vi "FocalMainV2.vi"() -> ()   [LabVIEW 2018]
uses:
  Clusters/FileDataChannel.ctl
  Clusters/BladePitchMode.ctl
  Clusters/GenMode.ctl
  Clusters/IndicatorScale.ctl
  Clusters/SimulationConstants.ctl
  Clusters/IOSignals.ctl
  <vilib>/Platform/TimedLoop/XDataNode/timing_clust.ctl
  <vilib>/Platform/TimedLoop/XDataNode/nitl_modes.ctl
  <vilib>/Platform/TimedLoop/XDataNode/wakeup.ctl
  Clusters/ArrayPairs.ctl
  Clusters/SwapArrayCluster.ctl
  Clusters/ElmoState.ctl
  Clusters/CtrlSignals.ctl
  Clusters/ScalingEnum.ctl
  Clusters/AnemometerData.ctl
  Clusters/RoscoParams.ctl
  Clusters/GenCtrl.ctl
  Clusters/PitchCtrl.ctl
  <vilib>/Instr/_visa.llb/VISA Configure Serial Port (Instr).vi
  SubVIs/InsertIntoArray_v2.vi
  <vilib>/platform/TimedLoop/XDataNode/XDataNode.xnode
  <vilib>/Platform/TimedLoop/XDataNode/XDNodeRunTimeDep.lvlib
  <resource>/objmgr/IndComECAT.rc
  usr/local/lib/libCallROSCO.so
  <vilib>/ptbypt/NI_PtbyPt.lvlib
panel:
  out "anemoRefU_m_s":dbl
  out "RS232 loop late?":bool
  in  "Fan Setpoint (%)":dbl format="%#_13g"
  out "Setpoint file loaded":path
  in  "Ctrl Mode":enum32{"Manual", "FromFile"}(radio)
  in  "Setpoint file name":string="setpointsVelTestA.txt"
  in  "Reload File":bool
  in  "windSpeed_m_s":dbl format="%#_13g"
  out "towerBotMy":dbl
  out "Current Setting":dbl[](array[numeric])
  in  "Commit":bool
  in  "Clear Faults":bool
  in  "Enable Fans":bool
  in  "Turn Fans On":bool
  out "Fy":dbl format="%#_5g"
  out "Fx":dbl
  out "PLC read errors":string
  out "PLC read/write late?":bool
  out "PLC Read Error":bool
  out "Axis 3 Homing":bool
  out "Axis 2 Homing":bool
  out "Axis 1 Homing":bool
  in  "Home Blades (x3)":bool
  out "Axis 3 Homed":bool
  out "Axis 2 Homed":bool
  out "Axis 1 Homed":bool
  out "SimulationConst":T1={"nGear"=1.0, "rotorRadius"=120.0, "numBlades"=3, "scaleFactor"=70.0, "roscoInitMinSpeed_rad_s"=0.5, "roscoInitMinTorqueFS_Nm"=1000000.0, "beckhoff16bit"=1000000.0, "beckhoff24BitExt"=7812500, "rotorTorqueScale_Nm_V"=5.0, "rotorTorqueOfst_Nm"=2.0, "rangeEL3104V"=10.0, "nacelleAccELM3604V"=1.25, "nacelleAccScaleX_m_s2_V"=0.0673, "nacelleAccOfstX_m_s2"=0.0055, "nacelleAccScaleY_m_s2_V"=0.0672, "nacelleAccOfstY_m_s2"=0.0049, "nacelleAccScaleZ_m_s2_V"=0.0677, "nacelleAccOfstZ_m_s2"=0.0087, "cyberGearRatio"=0.5, "cyberLinesPerRev"=0.5, "cyberRatedTorque"=0.5, "towerTopForceScale"=0.5, "towerTopTorqueScale"=0.5, "plcSetpointScaling_norm2VFD"=0.5, "towerBotScaleMy_Nm_V"=0.5, "towerBotOfstMy_Nm"=0.5, "towerTopScaleXaxis_N_V"=0.5, "towerTopOfstXaxis_N"=0.5, "towerTopScaleYaxis_N_V"=0.5, "towerTopOfstYaxis_N"=0.5, "pitchFlagOffset_deg"=0.5, "anemWindSpeedScaleU_m_s_m_s"=0.5, "anemWindSpeedOfstU_m_s"=0.5, "anemWindSpeedScaleV_m_s_m_s"=0.5, "anemWindSpeedOfstV_m_s"=0.5, "anemWindSpeedScaleW_m_s_m_s"=0.5, "anemWindSpeedOfstW_m_s"=0.5, "anemWindSpeedScaleTSI1_m_s_V"=0.5, "anemWindSpeedOfstTSI1_m_s"=0.5} {"beckhoff16bit" format="%x"}
  out "nacelleAccZ (m/s2)":dbl
  out "nacelleAccY (m/s2)":dbl
  out "nacelleAccX (m/s2)":dbl
  out "Disk > 2GB free?":bool
  out "Current OP mode":T2
  in  "IndicatorScale":T3
  in  "DISCON.IN file":string="DISCON-UMaineSemi.IN"
  in  "Cp/Ct/Cq file":string="Cp_Ct_Cq.IEA15MW.txt"
  out "Torque sine period FS (Nm)":dbl format="%.2g"
  out "Torque sine amp FS (Nm)":dbl format="%.2g"
  out "Torque sine mean FS (Nm)":dbl format="%.2g"
  out "Ramp time FS (s)":dbl format="%.2g"
  out "Ramp target vel FS (rpm)":dbl format="%.2g"
  out "Const. vel setpoint FS (rpm)":dbl format="%.2g"
  out "From File RotSpd FS (rpm)":dbl
  out "From File Pitch FS (deg)":dbl
  out "Exp time FS (s)":dbl format="%5.2f"
  in  "Commit gen settings":bool
  out "Current OP mode":T4
  in  "Commit pitch settings":bool
  in  "Start / Stop Run":bool
  out "Speed Setpoint (rpm)":dbl(knob)=7.068579725455493e-05 scale=0.0..20.0
  out "Pitch Blade 3 (deg)":dbl
  out "Pitch Bade 2 (deg)":dbl
  out "Pitch Blade 1 (deg)":dbl
  out "Pitch Setpoint (deg)":dbl
  out "Torque sine period MS (Nm)":dbl format="%.2g"
  out "Torque sine amp MS (Nm)":dbl format="%#.2g"
  in  "Torque sine period (s)":dbl=100.0
  in  "Torque sine amp (MNm)":dbl
  out "Torque sine mean MS (Nm)":dbl format="%.2g"
  in  "Torque mean (MNm)":dbl
  out "Ramp time MS (s)":dbl format="%.2g"
  out "Ramp target vel MS (rpm)":dbl format="%.2g"
  out "Const. vel setpoint MS (rpm)":dbl format="%.2g"
  in  "Ramp time (s)":dbl=100.0
  in  "Ramp target vel (rpm)":dbl=1.0
  in  "Const. vel (rpm)":dbl
  out "Current Const. (deg)":dbl
  in  "Next OP mode":T2
  in  "Next Const. (deg)":dbl=10.0
  in  "Next OP mode":T4
  in  "Wind Est. u(t=0)":dbl=5.0
  out "Exp. Time MS (s)":dbl format="%5.1f"
  out "Output file Name":string
  out "State logic late?":bool
  out "Axis 3 Fault":bool
  out "Axis 3 Warning":bool
  out "Axis 2 Fault":bool
  out "Axis 2 Warning":bool
  out "Axis 1 Fault":bool
  out "Axis 1 Warning":bool
  out "Axis 3 Operational":bool
  out "Axis 2 Operational":bool
  out "Axis 1 Operational":bool
  out "Pitch Axis 3 State":string
  out "Pitch Axis 2 State":string
  out "Pitch Axis 1 State":string
  in  "Clear Pitch Actuator Faults (x3)":bool
  in  "Enable Pitch Actuators (x3)":bool
  out "Generator Operational":bool
  in  "Clear Accelnet Faults":bool
  in  "Enable Accelnet":bool
  out "Generator Fault":bool
  out "Generator Warning":bool
  out "Main generator state":string
  out "Rosco Failed?":bool
  out "Torque Cell":dbl(knob) scale=0.0..25.0
  out "Actual Speed MS (rpm)":dbl(knob)=7.068579725455493e-05 scale=0.0..20.0
  in  "?":T5(tab)
  out "Accel":dynamicdata(graph)
  out "Generator Speed":dynamicdata(graph)
  out "Rotor Loads":dynamicdata(graph)
  out "Pitch":dynamicdata(graph)
  in  "Sample":bool
  in  "Apply Ofst":bool
  out "FxMean":dbl format="%0.2f"
  out "FyMean":dbl format="%0.2f"
  out "MyMean":dbl format="%0.2f"
  out "DISCON.IN Contents":string
  out "Rosco Interface Current Message":string
  out "ROSCO DISCON.In file used":string
  out "ROSCO CpCqCt File used":string
  out "ROSCO out file used":string
  out "Test sum":sgl
  out "error out":errorcluster
  out "aviFAIL":i32
  out "Rosco Interface First Message":string
  out "Rosco Setpoint (Nm) - MS":dbl(knob) scale=0.0..10.0
  out "OUT_ROTSP":dbl
  out "OUT_AEROTQ":dbl
  out "Rosco Pitch Setpoint (rad)":dbl(knob) scale=0.0..10.0
  out "WE ROSCO":dbl
  out "avrSWAP":sgl[](array[numeric])
  out "Setpoints":dbl[][](array[numeric])
  out "Time index":i32
  out "Loop duration (ms)":i64
  in  "Pitch Max Vel Change (rpm/min) - FS":dbl=10.0
  in  "Pitch Max Vel (rpm) - FS":dbl=1.0
  in  "Pitch Homing Vel  (rpm) - FS":dbl=0.3
  in  "Pitch P-Gain":dbl=5.0
  in  "Max Vel (rpm)  -FS":dbl=14.0
  in  "Velocity Ctrl P-Gain":dbl=0.14
  in  "Velocity Ctrl I-Gain":dbl=3.0
  in  "Torque Ctrl FF Gain":dbl=1.15
  in  "Torque Ctrl I-Gain":dbl=5.0
  in  "Torque Ctrl P-Gain":dbl=0.05
  in  "Max Torque (MNm) - FS":dbl=25.0
  out "Pitch axis 3 ctrl word":u16 format="%x"
  out "Pitch axis 2 ctrl word":u16 format="%x"
  out "RT Loop Duration":i64
  out "Control Mode - Main Gen":u8
  out "WriteSDO Abort - Main Gen":u32
  out "ReadSDO Abort - Main Gen":u32
  out "Gen ctrl word":u16 format="%x"
  out "Pitch axis 1 ctrl word":u16 format="%x"
  out "Graphics Update t (s)":dbl format="%.1f"
  out "Effective graphics rate (ms)":dbl format="%#.1f"
  out "WriteSDO Abort - Pitch 1":u32
  out "ReadSDO Abort - Pitch 1":u32
  out "Control Mode - Pitch 1":u8
  out "Torque RAW (V)":dbl
  out "Torque Sensor (Nm) - NOT scaled":dbl(knob) scale=-2.0..2.0
  out "Free GB disk":dbl
  out "WriteSDO Abort - Pitch 2":u32
  out "Control Mode - Pitch 2":u8
  out "ReadSDO Abort - Pitch 2":u32
  out "WriteSDO Abort - Pitch 3":u32
  out "Control Mode - Pitch 3":u8
  out "ReadSDO Abort - Pitch 3":u32
  out "MotorDemandTorque_Nm":dbl(knob) scale=-2.0..2.0
  out "MotorCurrentTorq (Nm)":dbl(knob) scale=-2.0..2.0
  out "Axis 1 HomePos (rad)":dbl
  out "Axis 2 HomePos (rad)":dbl
  out "Axis 3 HomePos (rad)":dbl
  out "Init error":errorcluster
  out "Setpoint read error":string
  out "Torque Setpoint":dbl(knob) scale=0.0..35.0
  out "Power (MW)":dbl(slide) scale=0.0..10.0 scale format="%.2f"
  out "FIFO Loop Late?":bool
  in  "Base filename":string="rosco-tests"
  out "Writing":bool
  in  "?":T6
  out "#RT FIFO":u32
  in  "Stop LabVIEW":bool
  out "cRio Time(s)":dbl format="%6.1f"
  out "RT Loop Late?":bool
  # "FOCAL Campaign 1 - V2.1"
  # "ROSCO OK?"
  # "GENERATOR ENABLE"
  # "BLADE PITCH"
  # "WIND MACHINE CONTROL"
  # "EXPERIMENT CONTROL"
  # "GENERATOR SETPOINT CTRL"
  # "PITCH ACTUATORS CONTROL"
  # "Nacelle Acceleration"
  # "TowerTop 3DOF"
  # "Blade1"
  # "Blade2"
  # "Blade3"
  # "Current values"
  # "Operational"
  # "Enter NEXT values (FS)"
  # "FS"
  # "MS"
  # "Homing"
  # "Homed"
  # "Warning"
  # "Error"
  # "TowerBot My"
  # "Fan 1"
  # "Time"
  # "Pitch"
  # "RotSpd"
  # "Fan 20"
  # "Fan 30"
  # "Fan 10"
  # "PI for Torque Ctrl"
  # "PI for Velocity Ctrl"
  # "PI for Pitch Ctrl"
  # "Main Gen Limits"
  # "Pitch limits"
  # "PITCH AXIS 1"
  # "PITCH AXIS 2"
  # "PITCH AXIS 3"
  # "TOWER TOP 6DOF"
  # "SYSTEM"
  # "GENERATOR"
  # "TORQUE SENSOR"
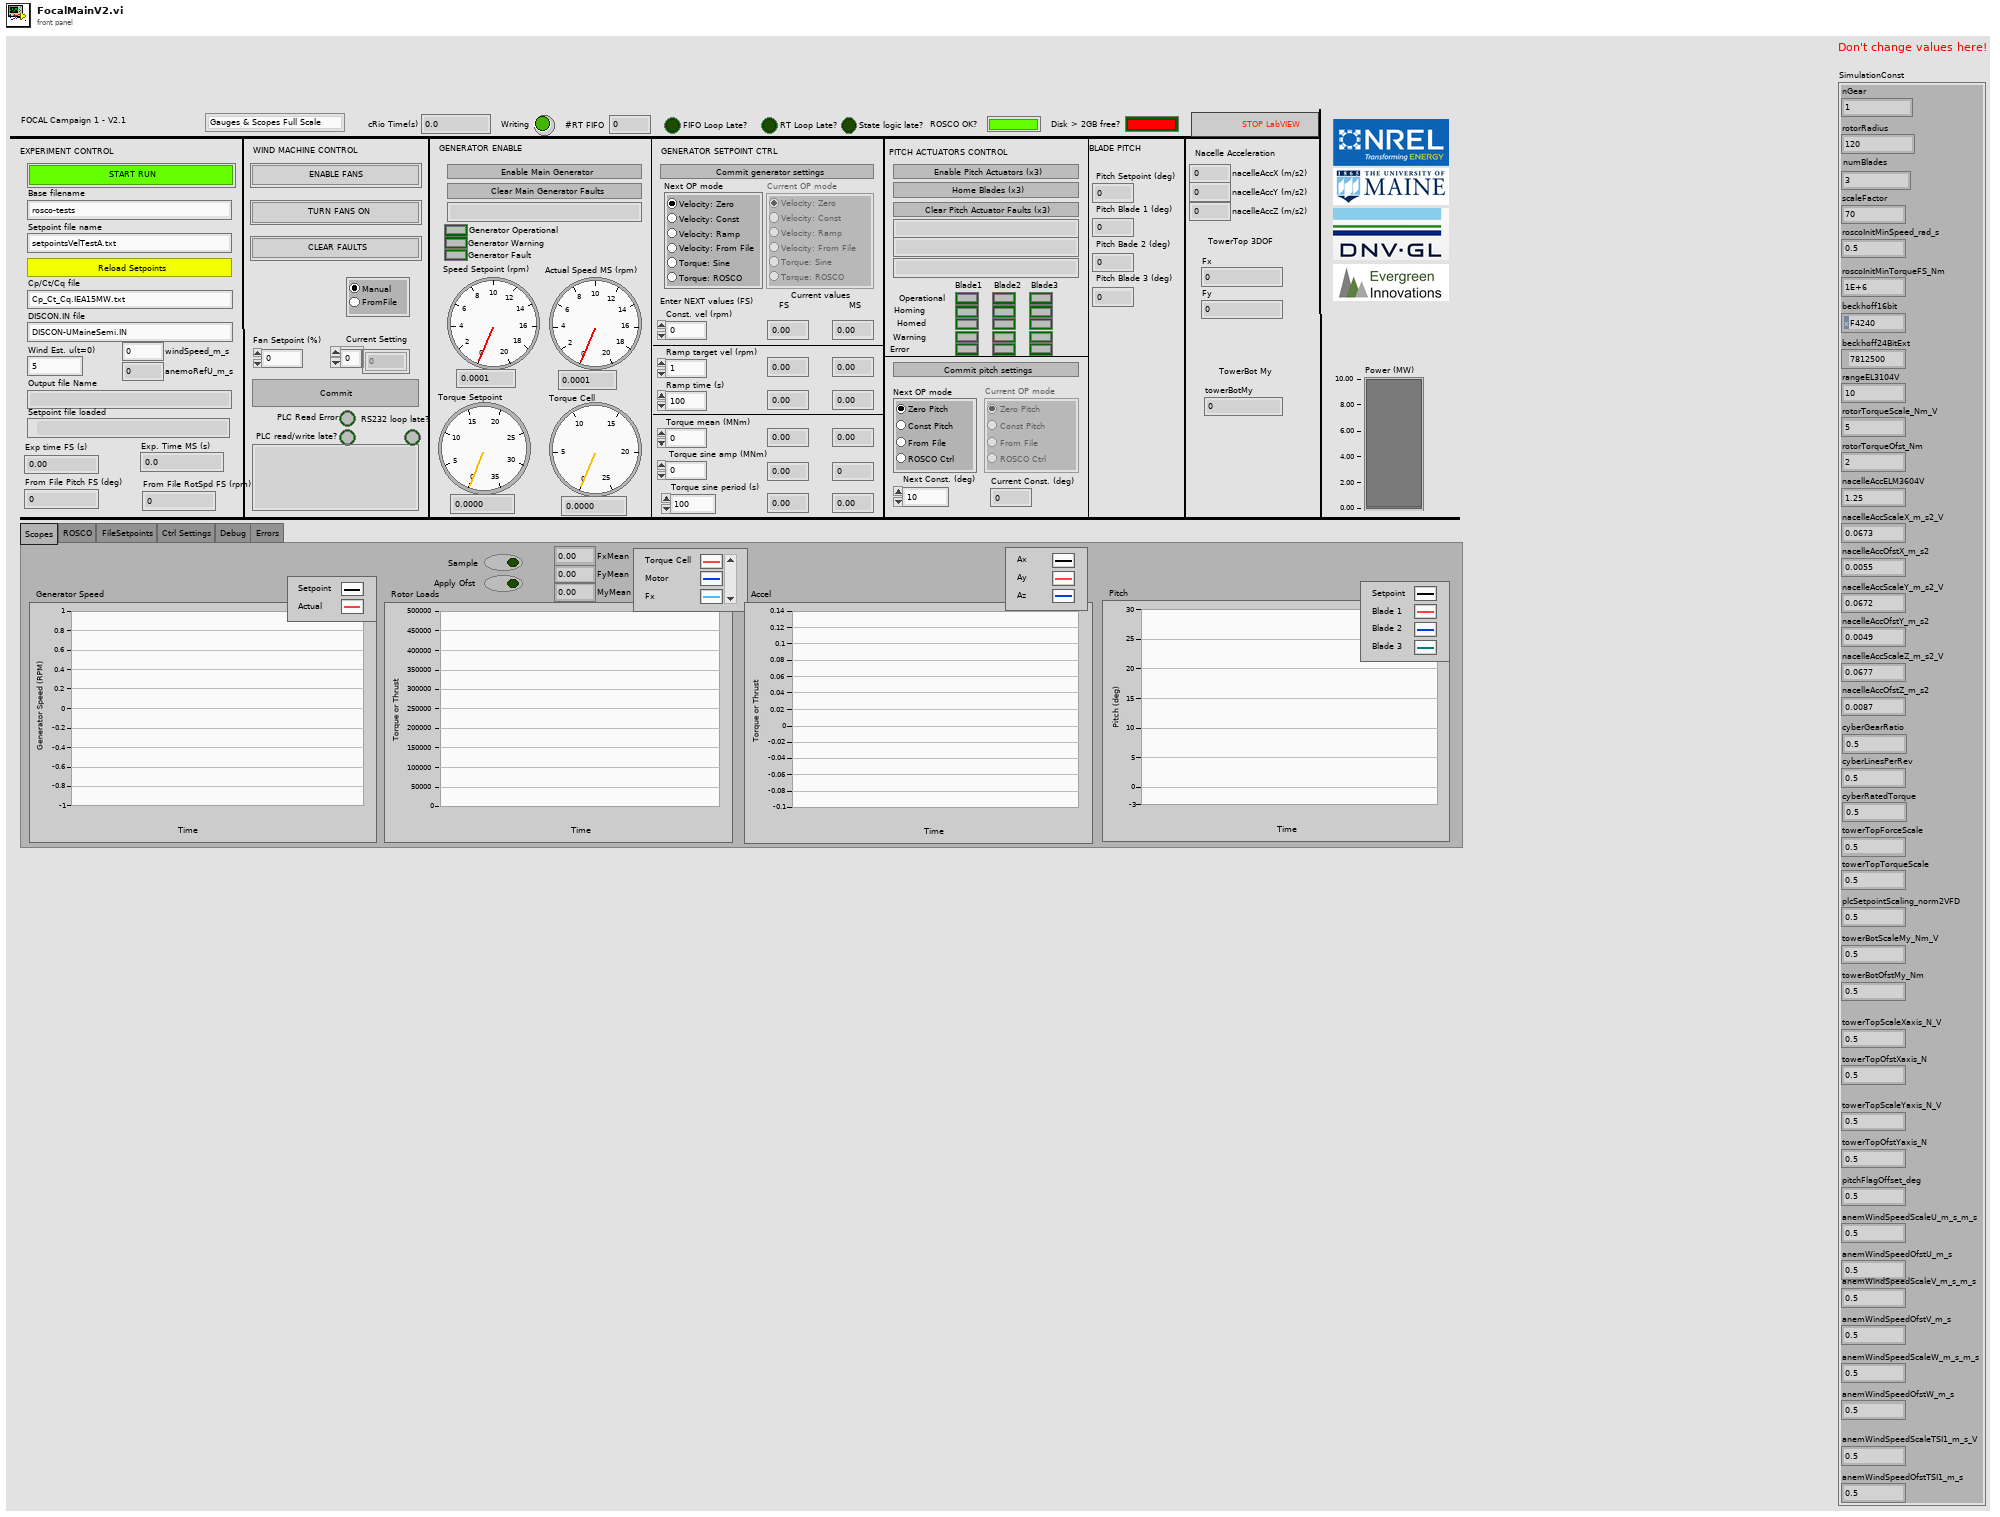
[diagram p1: front panel]
types:
  T1 = typedef "SimulationConstants.ctl" = cluster{"nGear":dbl, "rotorRadius":sgl, "numBlades":i32, "scaleFactor":dbl, "roscoInitMinSpeed_rad_s":dbl, "roscoInitMinTorqueFS_Nm":dbl, "beckhoff16bit":dbl, "beckhoff24BitExt":i32, "rotorTorqueScale_Nm_V":dbl, "rotorTorqueOfst_Nm":dbl, "rangeEL3104V":dbl, "nacelleAccELM3604V":dbl, "nacelleAccScaleX_m_s2_V":dbl, "nacelleAccOfstX_m_s2":dbl, "nacelleAccScaleY_m_s2_V":dbl, "nacelleAccOfstY_m_s2":dbl, "nacelleAccScaleZ_m_s2_V":dbl, "nacelleAccOfstZ_m_s2":dbl, "cyberGearRatio":dbl, "cyberLinesPerRev":dbl, "cyberRatedTorque":dbl, "towerTopForceScale":dbl, "towerTopTorqueScale":dbl, "plcSetpointScaling_norm2VFD":dbl, "towerBotScaleMy_Nm_V":dbl, "towerBotOfstMy_Nm":dbl, "towerTopScaleXaxis_N_V":dbl, "towerTopOfstXaxis_N":dbl, "towerTopScaleYaxis_N_V":dbl, "towerTopOfstYaxis_N":dbl, "pitchFlagOffset_deg":dbl, "anemWindSpeedScaleU_m_s_m_s":dbl, "anemWindSpeedOfstU_m_s":dbl, "anemWindSpeedScaleV_m_s_m_s":dbl, "anemWindSpeedOfstV_m_s":dbl, "anemWindSpeedScaleW_m_s_m_s":dbl, "anemWindSpeedOfstW_m_s":dbl, "anemWindSpeedScaleTSI1_m_s_V":dbl, "anemWindSpeedOfstTSI1_m_s":dbl}
  T2 = typedef "GenMode.ctl" = enum32{"Velocity: Zero", "Velocity: Const.", "Velocity: Ramp", "Velocity: From File", "Torque: Sine", "Torque: ROSCO"}
  T3 = typedef "IndicatorScale.ctl" = enum16{"Gauges & Scopes Full Scale", "Gauges & Scopes Model Scale"}
  T4 = typedef "BladePitchMode.ctl" = enum32{"Zero pitch", "Const pitch", "From File", "ROSCO Ctrl"}
  T5 = enum32{"Scopes", "ROSCO", "FileSetpoints", "Ctrl Settings", "Debug", "Errors"}
  T6 = typedef "FileDataChannel.ctl" = cluster{"dataTime_s":dbl, "dataLoopCounter":dbl, "anemoRefU_m_s":dbl, "anemoRefV_m_s":dbl, "anemoRefW_m_s":dbl, "rotorTorque_Nm":dbl, "towerTopFx_N":dbl, "towerTopFy_N":dbl, "towerBotMy_Nm":dbl, "accelNacelleAx_m_s2":dbl, "accelNacelleAy_m_s2":dbl, "accelNacelleAz_m_s2":dbl, "genSpeed_rad_s":dbl, "genTorque_Nm":dbl, "genStatus":dbl, "pitch1Position_rad":dbl, "pitch1Velocity_rad_s":dbl, "pitch1Status":dbl, "pitch2Position_rad":dbl, "pitch2Velocity_rad_s":dbl, "pitch2Status":dbl, "pitch3Position_rad":dbl, "pitch3Velocity_rad_s":dbl, "pitch3Status":dbl, "genUserOpMode":dbl, "pitchUserOpMode":dbl, "torqueSetpointRosco_Nm":dbl, "pitchSetpointRosco_rad":dbl, "fan1Setpt_%":dbl, "genTorqueSetpointActual_Nm":dbl, "pitchSetpointActual_rad":dbl, "genVelSetpoint_radps":dbl, "genPosition_rad":dbl, "towerTopFz_N":dbl, "towerTopMx_Nm":dbl, "towerTopMy_Nm":dbl, "towerTopMz_Nm":dbl}
  T7 = typedef "CtrlSignals.ctl" = cluster{"Enable":bool, "On":bool, "Reset Fault":bool}
  T8 = typedef "ElmoState.ctl" = cluster{"Elmo Operational":bool, "Elmo Warning":bool, "Elmo Fault":bool, "Blade Homed":bool, "Blade Homing":bool, "HomePos (rad)":dbl}
  T9 = typedef "ArrayPairs.ctl" = cluster{"iStatus":T10, "TIME":T10, "DT":T10, "Blade1PitchPos_rad":T10, "VS_MECHGENPWR":T10, "VS_GENPWR":T10, "GEN_SPEED":T10, "ROTOR_SPEED":T10, "GENTQMEAS":T10, "Y_M":T10, "HORWINDV":T10, "ROOTMOOP1":T10, "ROOTMOOP2":T10, "Blade2PitchPos_rad":T10, "Blade3PitchPos_rad":T10, "ROOTMOOP3":T10, "AVCMSG_SIZE":T10, "INFILE_SIZE ":T10, "OUTFILE_SIZE ":T10, "FA_ACC":T10, "NUM_BLADES":T10, "BladePitchSetpoint_rad":T10, "TorqueSetpoint_Nm":T10, "OUT_AEROTQ":T10, "Out.RotSpeed ":T10, "Out.DEBUG":T10}
  T10 = typedef "SwapArrayCluster.ctl" = cluster{"Index":i32, "Value":dbl}
  T11 = typedef "IOSignals.ctl" = cluster{"mainGenPosition (rad)":dbl, "motorCurrentTorq (Nm)":dbl, "mainGenVelocity (rad/s)":dbl, "mainGenStatus":u16, "pitch1Position (rad)":dbl, "pitch1Velocity (rad/s)":dbl, "pitch1Status":u16, "pitch2Position (rad)":dbl, "pitch2Velocity (rad/s)":dbl, "pitch2Status":u16, "pitch3Position (rad)":dbl, "pitch3Velocity (rad/s)":dbl, "pitch3Status":u16, "torqueSensor (Nm)":dbl, "nacelleAccX (m/s2)":dbl, "nacelleAccY (m/s2)":dbl, "nacelleAccZ (m/s2)":dbl, "pitch1HomeFlag":bool, "pitch2HomeFlag":bool, "pitch3HomeFlag":bool, "towerTopFx (N)":dbl, "towerTopFy (N)":dbl, "towerBotMy (Nm)":dbl, "anemoRefU_m_s":dbl, "anemoRefV_m_s":dbl, "anemoRefW_m_s":dbl}
  T12 = enum16{"open", "replace", "create", "open or create", "replace or create", "replace or create with confirmation"}
  T13 = typedef "RoscoParams.ctl" = cluster{"avrSWAP":dbl[], "aviFAIL":i32, "currentMsg":string, "ReturnValue":i32, "disconInFileName":string, "outFileName":string, "firstMsg":string}
  T14 = typedef "XDNodeRunTimeDep.lvlib/timing_clust.ctl" = cluster{"Expected End [f-1]":u64, "Actual End [f-1]":u64, "Finished Late? [f-1]":bool, "Expected End [i-1]":u64, "Actual End [i-1]":u64, "Finished Late? [i-1]":bool, "Expected Start [i]":u64, "Actual Start [i]":u64, "Expected Start [f]":u64, "Actual Start [f]":u64, "Source Name":string, "Structure Name":string, "Period":i64, "Deadline":i64, "Offset":i64, "Start":i64, "Priority":i32, "Timeout":i32, "Mode":T15, "Wakeup Reason":T16, "Error":errorcluster, "Source Type":string, "Secondary Source Type":string, "Global End Time":u64, "Global Start Time":u64, "Frame Duration":u64, "Iteration Duration":u64, "Assigned CPU":i32, "I/O Scan Engine Mode":u32}
  T15 = typedef "XDNodeRunTimeDep.lvlib/nitl_modes.ctl" = enum32{"No Change", "Process missed periods, maintain original phase", "Discard missed periods, maintain original phase", "Process missed periods, ignore original phase", "Discard missed periods, ignore original phase"}
  T16 = typedef "XDNodeRunTimeDep.lvlib/wakeup.ctl" = enum32{"Normal", "Aborted", "Asynchronous wakeup", "Timing source error", "Timed loop error", "Timeout"}
  T17 = enum8{"Enabled", "Disabled", "Disabled and Grayed Out"}
  T18 = typedef "ScalingEnum.ctl" = enum16{"Model scale -> Full scale", "Full scale -> Model scale"}
  T19 = typedef "GenCtrl.ctl" = cluster{"Constant velocity setpoint (rpm)":dbl, "Ramp target velocity (rpm)":dbl, "Ramp time (s)":dbl, "Sine mean (Nm)":dbl, "Sine amp (Nm)":dbl, "Sine period (s)":dbl, "Torque Ctrl I-Gain":dbl, "Velocity Ctrl P-Gain":dbl, "Velocity Ctrl I-Gain":dbl, "Max Torque (Nm)":dbl, "GeneratorOn":bool, "Torque Ctrl P-Gain":dbl, "From file velocity (rpm)":dbl, "Generator operating mode":T2, "Max Vel (rpm)":dbl, "Torque Ctrl FF Gain":dbl}
  T20 = typedef "PitchCtrl.ctl" = cluster{"P-Gain":dbl, "Blade pitch operating mode":T4, "Constant setpoint (deg)":dbl, "I-Gain":dbl, "Pitch from File (deg)":dbl, "Homing vel (rpm)":dbl, "Max vel (rpm)":dbl, "Max vel change (rpm/min)":dbl}
  T21 = typedef "AnemometerData.ctl" = cluster{"Wind speed, U (m/s)":dbl, "Wind speed, V (m/s)":dbl, "Wind speed, W (m/s)":dbl}
  T22 = typedef "AccelnetState.ctl" = cluster{"State String":string, "Accelnet Warning":bool, "Accelnet Fault":bool, "Accelnet Operational":bool}
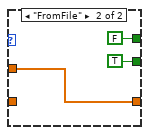
[diagram p5: hidden frame]
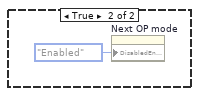
[diagram p12: hidden frame]
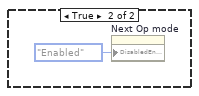
[diagram p13: hidden frame]
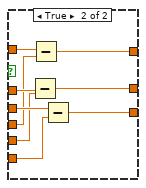
[diagram p15: hidden frame]
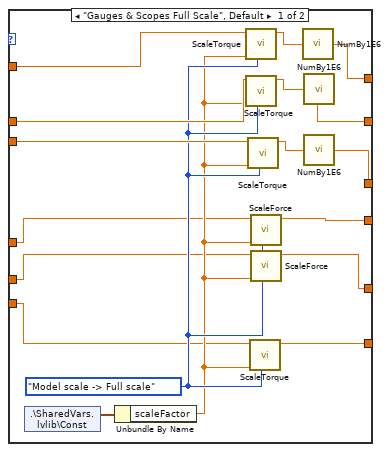
[diagram p17: hidden frame]
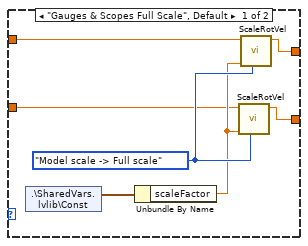
[diagram p18: hidden frame]
diagram:
  w2 = T7 {"Enable"=FALSE, "On"=FALSE, "Reset Fault"=FALSE}  # Ctrl State
  w10 = T7 {"Enable"=FALSE, "On"=FALSE, "Reset Fault"=FALSE}  # Current State
  w8 = errorcluster {"status"=FALSE, "code"=0, "source"=""}  # Error
  w20 = u16 10 items=["1.0"=10, "1.5"=15, "2.0"=20] ("stop bits (10: 1 bit)")
  w21 = u16 0 items=["None", "XON/XOFF", "RTS/CTS", "XON/XOFF & RTS/CTS", "DTR/DSR", "XON/XOFF & DTR/DSR"] ("flow control (0:none)")
  w74 = i64 2000 ("Period")
  # "Setpoint VFD"
  # "Current VFD read from PLC"
  # "Adjust this once we get a feeling for IO latency to/from the PLC"
  # "Runs at 64 Hz = 15.625ms = 15625 us"
  # "Manual Vel Set"
  # "Rotor Spd init"
  # "Blade Pitch init"
  # "Velocity Setpoint init"
  # "Time init"
  # "us -> s"
  # "in us"
  # "Init torque sine period"
  # "Init torque sine amp"
  # "Init torque mean"
  # "Init Ramp time"
  # "Init Ramp target vel"
  # "Init Const. Vel"
  # "Initial pitch"
  # "Code to remove"
  # "dt (s)"
  # "5ms = 200Hz"
  # "group name"
  n1 = flat-sequence {
    tunnel: [w123] -> w89
    tunnel: [w124] -> w88
    tunnel: [w116] -> w82
    tunnel: [w115] -> w81
    tunnel: [w102] -> w54
    tunnel: [w101] -> w53
    tunnel: [w100] -> w52
    tunnel: [w99] -> w51
    tunnel: w89 -> [w167]
    tunnel: w88 -> [w166]
    tunnel: w82 -> [w157]
    tunnel: w81 -> [w156]
    tunnel: [w153] -> w48
    tunnel: w54 -> [w144]
    tunnel: w53 -> [w143]
    tunnel: w52 -> [w133]
    tunnel: w51 -> [w132]
    tunnel: w48 -> [w177]
    tunnel: [w177] -> w47
    tunnel: [w225] -> w84
    tunnel: [w219] -> w92
    tunnel: [w212] -> w67
    tunnel: w47 -> [w212]
    tunnel: [w193] -> w56
    frame #0 {
      w100 = refnum<k21> "ni.var.io://NI-cRIO-9036-01B82934/EtherCAT Master/PitchBlade3" ("Slave Constant")
      w102 = refnum<k21> "ni.var.io://NI-cRIO-9036-01B82934/EtherCAT Master/PitchBlade2" ("Slave Constant")
      w116 = refnum<k21> "ni.var.io://NI-cRIO-9036-01B82934/EtherCAT Master/PitchBlade1" ("Slave Constant")
      w123 = refnum<k21> "ni.var.io://NI-cRIO-9036-01B82934/EtherCAT Master/MainGen" ("Slave Constant")
      # "Mode of operation for Pitch Blade 3"
      # "Mode of operation"
      # "8 = CSP \n9 = CSV\n10 = CST"
      # "Mode of operation for Pitch Blade 2"
      # "Mode of operation"
      # "8 = CSP \n9 = CSV\n10 = CST"
      # "Note: Operate in CST, and close velocity loop in LabVIEW when required"
      # "Mode of operation for Pitch Blade 1"
      # "Mode of operation for Main Gen"
      # "Mode of operation"
      # "8 = CSP \n9 = CSV\n10 = CST"
      # "Mode of operation"
      # "9 = CSV\n10 = CST"
      # "Set modes of operation for main generator and pitch actuators"
      n2 = invoke class="IndComECAT Slave" method="neLVRefNum_Slave_WriteSDO"(reference=w116, "Blocking"=TRUE, "OD Addr"=u16 0, "Index"=u16 24672, "Subindex"=u8 0, "Data"=u8[] [9]) -> (error out=w115:errorcluster, "Abort Code"=→"WriteSDO Abort - Pitch 1":u32)  [unwired: 3 in, 7 out]
      n3 = invoke class="IndComECAT Slave" method="neLVRefNum_Slave_WriteSDO"(reference=w102, "Blocking"=TRUE, "OD Addr"=u16 0, "Index"=u16 24672, "Subindex"=u8 0, "Data"=u8[] [9]) -> (error out=w101:errorcluster, "Abort Code"=→"WriteSDO Abort - Pitch 2":u32)  [unwired: 3 in, 7 out]
      n4 = invoke class="IndComECAT Slave" method="neLVRefNum_Slave_WriteSDO"(reference=w123, "Blocking"=TRUE, "OD Addr"=u16 0, "Index"=u16 24672, "Subindex"=u8 0, "Data"=u8[] [9]) -> (error out=w124:errorcluster, "Abort Code"=→"WriteSDO Abort - Main Gen":u32)  [unwired: 3 in, 7 out]
      n5 = invoke class="IndComECAT Slave" method="neLVRefNum_Slave_WriteSDO"(reference=w100, "Blocking"=TRUE, "OD Addr"=u16 0, "Index"=u16 24672, "Subindex"=u8 0, "Data"=u8[] [9]) -> (error out=w99:errorcluster, "Abort Code"=→"WriteSDO Abort - Pitch 3":u32)  [unwired: 3 in, 7 out]
    }
    frame #1 {
      # "Mode of operation"
      # "Mode of operation"
      # "Mode of operation"
      # "Mode of operation"
      # "Check generator and pitch actuator control modes"
      n6 = invoke class="IndComECAT Slave" method="neLVRefNum_Slave_ReadSDO"(reference=w167, error in=w166, "blocking"=TRUE, "odAddr"=u16 0 ("OD address"), "index"=u16 24672 ("Index"), "subIndex"=u8 0 ("Subindex")) -> (error out=w155:errorcluster, "data"=w170:u8[], "abortCode"=→"ReadSDO Abort - Main Gen":u32)  [unwired: 3 in, 6 out]
      n7 = invoke class="IndComECAT Slave" method="neLVRefNum_Slave_ReadSDO"(reference=w144, error in=w143, "blocking"=TRUE, "odAddr"=u16 0 ("OD address"), "index"=u16 24672 ("Index"), "subIndex"=u8 0 ("Subindex")) -> (error out=w142:errorcluster, "data"=w150:u8[], "abortCode"=→"ReadSDO Abort - Pitch 2":u32)  [unwired: 3 in, 6 out]
      n8 = invoke class="IndComECAT Slave" method="neLVRefNum_Slave_ReadSDO"(reference=w133, error in=w132, "blocking"=TRUE, "odAddr"=u16 0 ("OD address"), "index"=u16 24672 ("Index"), "subIndex"=u8 0 ("Subindex")) -> (error out=w131:errorcluster, "data"=w136:u8[], "abortCode"=→"ReadSDO Abort - Pitch 3":u32)  [unwired: 3 in, 6 out]
      n9 = invoke class="IndComECAT Slave" method="neLVRefNum_Slave_ReadSDO"(reference=w157, error in=w156, "blocking"=TRUE, "odAddr"=u16 0 ("OD address"), "index"=u16 24672 ("Index"), "subIndex"=u8 0 ("Subindex")) -> (error out=w154:errorcluster, "data"=w160:u8[], "abortCode"=→"ReadSDO Abort - Pitch 1":u32)  [unwired: 3 in, 6 out]
      n10 = Index Array(array=w170, index=0) -> (element=→"Control Mode - Main Gen":u8)
      n11 = Index Array(array=w150, index=0) -> (element=→"Control Mode - Pitch 2":u8)
      n12 = Index Array(array=w136, index=0) -> (element=→"Control Mode - Pitch 3":u8)
      n13 = Index Array(array=w160, index=0) -> (element=→"Control Mode - Pitch 1":u8)
      n14 = Merge Errors(w155, w154, w142, w131) -> (w153:errorcluster)
    }
    frame #2 {
      w176 = T1 {"nGear"=1.0, "rotorRadius"=120.0, "numBlades"=3, "scaleFactor"=70.0, "roscoInitMinSpeed_rad_s"=0.5, "roscoInitMinTorqueFS_Nm"=1000000.0, "beckhoff16bit"=32768.0, "beckhoff24BitExt"=7812500, "rotorTorqueScale_Nm_V"=1.0, "rotorTorqueOfst_Nm"=-0.02, "rangeEL3104V"=10.0, "nacelleAccELM3604V"=1.25, "nacelleAccScaleX_m_s2_V"=14.859, "nacelleAccOfstX_m_s2"=0.081724, "nacelleAccScaleY_m_s2_V"=14.881, "nacelleAccOfstY_m_s2"=0.072917, "nacelleAccScaleZ_m_s2_V"=14.771, "nacelleAccOfstZ_m_s2"=0.128508, "cyberGearRatio"=64.0, "cyberLinesPerRev"=4096.0, "cyberRatedTorque"=5.1, "towerTopForceScale"=1000000.0, "towerTopTorqueScale"=1000000.0, "plcSetpointScaling_norm2VFD"=6000.0, "towerBotScaleMy_Nm_V"=193147.3, "towerBotOfstMy_Nm"=-0.0109, "towerTopScaleXaxis_N_V"=93217.84, "towerTopOfstXaxis_N"=-1.19319, "towerTopScaleYaxis_N_V"=88458.94, "towerTopOfstYaxis_N"=1.362268, "pitchFlagOffset_deg"=-4.0, "anemWindSpeedScaleU_m_s_m_s"=1.0, "anemWindSpeedOfstU_m_s"=0.0, "anemWindSpeedScaleV_m_s_m_s"=1.0, "anemWindSpeedOfstV_m_s"=0.0, "anemWindSpeedScaleW_m_s_m_s"=1.0, "anemWindSpeedOfstW_m_s"=0.0, "anemWindSpeedScaleTSI1_m_s_V"=1.0, "anemWindSpeedOfstTSI1_m_s"=0.0} ("SimulationConst")
      # "Note:\nnacelleAcc constants are inverted (1/x) from manufacturer sheets due to how we apply scale\nConstants are applied based on sensor channel, not basin coordinate system. \nAny change in sign is done in readIO to assign the correct channels and orientation\n\nReference Calibrations_Summary_DATE.xlsx"
      # "Define constants to be used in the code"
      # "Define constants"
      n15 = shared-variable ".\\SharedVars.lvlib\\Const"(w176) -> ()  [unwired: 1 in, 1 out]
      "SimulationConst" <- w176
    }
    frame #3 {
      w205 = path "C:/rosco-data" ("path")
      # "This file will be picked up via DISCON.IN / ROSCO"
      # "Checks if DISCON.IN exists"
      # "Allocate memory for ROSCO return message"
      # "Up to 500 entries in SWAP array"
      # "No. of buffer slices"
      # "This is the typedef for File IO"
      # "number of channels"
      # "Read required files and initialize various arrays"
      n16 = disable-structure shown="Disabled" {
        frame Disabled {
          # "Note: DO NOT run this code in normal operation. Will  cause the .so file to not unload properly."
          # "Test function into libCallROSCO"
          n17 = dll-call lib="usr/local/lib/libCallROSCO.so" fn="add"("a"=sgl 1.0, "b"=sgl 8.0) -> (error out=→"error out":errorcluster, "sum"=→"Test sum":sgl)  [unwired: 5 in, 1 out]
        }
        frame Enabled {
        }
      }
      n18 = property on="Base filename" class="Str"("Value"="focal_series_000" ("Base filename")) -> ()  [unwired: 2 in, 2 out]
      n19 = property on="Rosco Interface Current Message" class="Str"("Value"="") -> ()  [unwired: 2 in, 2 out]
      n20 = property on="Base filename" class="Str"("Value"="") -> ()  [unwired: 2 in, 2 out]
      n21 = property on="StopLabVIEW" class="Bool (strict)"("Value"=FALSE) -> ()  [unwired: 2 in, 2 out]
      n22 = property on="Enable Accelnet" class="Bool (strict)"("Value"=FALSE ("Enable Accelnet")) -> ()  [unwired: 2 in, 2 out]
      n23 = property on="Enable Pitch Actuators (x3)" class="Bool (strict)"("Value"=FALSE ("Enable Pitch Actuators (x3)")) -> ()  [unwired: 2 in, 2 out]
      n24 = property on="Next Op mode" class="RadioBtnsControl (strict)"("Value"=GenMode."Velocity: Zero" ("Next Op mode")) -> ()  [unwired: 2 in, 2 out]
      n25 = property on="Next OP mode" class="RadioBtnsControl (strict)"("Value"=BladePitchMode."Zero pitch" ("Next OP mode")) -> ()  [unwired: 2 in, 2 out]
      n26 = Build Path(base path=w205, name or relative path="roscoOut.txt") -> (appended path=w203:path)
      n27 = Build Path(base path=w205, name or relative path="Cp/Ct/Cq file") -> (appended path=w210:path)
      n28 = Build Path(base path=w205, name or relative path="DISCON.IN file") -> (appended path=w206:path)
      n29 = call "ConfigFileExists.vi"("Path   In"=w206) -> ("Path Out"=w199:path)  [unwired: 9 in, 1 out]
      n30 = call "ConfigFileExists.vi"("Path   In"=w210) -> ("Path Out"=w209:path)  [unwired: 9 in, 1 out]
      n31 = Path To String(path=w203) -> (string=w202:string)
      "ROSCO out file used" <- w202
      n32 = Path To String(path=w209) -> (string=→"ROSCO CpCqCt File used":string)
      n33 = Path To String(path=w199) -> (string=w201:string)
      "ROSCO DISCON.In file used" <- w201
      n34 = Open/Create/Replace File(file path (use dialog)=w199, operation (0:open)=T12."open") -> (refnum out=w197:refnum<file>, error out=w200:errorcluster)  [unwired: 4 in, 1 out]
      n35 = property on="Velocity Ctrl P-Gain" class="DigNum (strict)"("Value"=0.05 ("Velocity Ctrl P-Gain")) -> ()  [unwired: 2 in, 2 out]
      n36 = property on="Velocity Ctrl I-Gain" class="DigNum (strict)"("Value"=7.0 ("Velocity Ctrl I-Gain")) -> ()  [unwired: 2 in, 2 out]
      n37 = property on="Max Torque (MNm) - FS" class="DigNum (strict)"("Value"=25.0 ("Max Torque (MNm) - FS")) -> ()  [unwired: 2 in, 2 out]
      n38 = property on="Max Vel (rpm)  -FS" class="DigNum (strict)"("Value"=15.0 ("Max Vel (rpm)  -FS")) -> ()  [unwired: 2 in, 2 out]
      n39 = property on="Torque Ctrl P-Gain" class="DigNum (strict)"("Value"=0.05 ("Torque Ctrl P-Gain")) -> ()  [unwired: 2 in, 2 out]
      n40 = property on="Torque Ctrl I-Gain" class="DigNum (strict)"("Value"=10.0 ("Torque Ctrl I-Gain")) -> ()  [unwired: 2 in, 2 out]
      n41 = property on="Torque Ctrl FF Gain" class="DigNum (strict)"("Value"=1.25 ("Torque Ctrl FF Gain")) -> ()  [unwired: 2 in, 2 out]
      n42 = call "StringInit.vi"("accOUTNAME"="First Msg", "dimension size"=8192) -> ("result string"=w189:string)  [unwired: 9 in]
      n43 = call "StringInit.vi"("accOUTNAME"="Current Msg", "dimension size"=8192) -> ("result string"=w192:string)  [unwired: 9 in]
      n44 = Initialize Array(0.0 ("element"), 500 ("dimension size")) -> (w217:dbl[])
      n45 = Read from Text File(file (use dialog)=w197, error in=w200) -> (refnum out=w195:refnum<file>, text=→"DISCON.IN Contents":string, error out=w194:errorcluster)  [unwired: 2 in, 1 out]
      n46 = Close File(refnum=w195, error in=w194) -> (error out=w193:errorcluster)  [unwired: 1 out]
      n47 = Bundle By Name(cluster=T13 {"avrSWAP"=[], "aviFAIL"=0, "currentMsg"="", "ReturnValue"=0, "disconInFileName"="", "outFileName"="", "firstMsg"=""}, "avrSWAP"=w217, "aviFAIL"=-100, "currentMsg"=w192, "firstMsg"=w189, "outFileName"=w202, "disconInFileName"=w201) -> (w219:T13)
      n48 = Cluster To Array(cluster="?") -> (array=w215:dbl[])
      n49 = Array Size(array=w215) -> (size(s)=w214:i32)
      n50 = To Unsigned Long Integer(number=w214) -> (unsigned 32bit integer=w213:u32)
      n51 = RT FIFO Create(0:"DataBuffer" ("name (unnamed)"), 1:dbl[] [] ("appended array"), 4:u32 200, 6:w213) -> (8:w225:refnum<k33>)  [unwired: 4 in, 2 out]
    }
  }
  n52 = disable-structure shown="Disabled" {
    frame Disabled {
      n53 = shared-variable ".\\SharedVars.lvlib\\SIM-GenSpeed_rad_s"(0.009999999776482582 ("RotorSpeed(rad/s)")) -> ()  [unwired: 1 in, 1 out]
      n54 = shared-variable ".\\SharedVars.lvlib\\SIM-BladePitch_rad"(0.0 ("ecat-BladePitch")) -> ()  [unwired: 1 in, 1 out]
      n55 = shared-variable ".\\SharedVars.lvlib\\SIM-WindSpeed_m_s"(0.0 ("WindSpeedSim")) -> ()  [unwired: 1 in, 1 out]
    }
    frame Enabled {
    }
  }
  n56 = disable-structure shown="Disabled" {
    frame Disabled {
      n57 = local read "DISCON.IN Contents"() -> ()  [unwired: 1 in]
    }
    frame Enabled {
    }
  }
  n58 = Merge Errors(w56, w67) -> (→"Init error":errorcluster)
  n59 = property on="SimulationConst" class="Clust (strict)"() -> ("Controls[]"=w46:refnum<vi>[])  [unwired: 2 in, 2 out]
  n60 = for {
    tunnel: w46 -> [w243] mode=indexing
    tunnel: [w244] -> w50 mode=indexing
    tunnel: [w240] -> w49 mode=indexing
    n61 = property class="Ctl"(reference=w243) -> ("Value"=w242:variant)  [unwired: 1 in, 2 out]
    n62 = property class="Ctl"(reference=w243) -> ("Label.Text"=w244:string)  [unwired: 1 in, 2 out]
    n63 = Variant To Data(type=0.0, Variant=w242) -> (data=w240:dbl)  [unwired: 1 in, 1 out]
  }
  n64 = Tick Count (ms)() -> (millisecond timer value=w83:u32)
  n65 = property class="Clust (strict)"() -> ("Controls[]"=w98:refnum<vi>[])  [unwired: 2 in, 2 out]
  n66 = To Double Precision Float(number=w74) -> (double precision float=w73:dbl)
  n67 = call-poly "VISA Configure Serial Port"("VISA resource name"=refnum<visa-resource-name> "ASRL1::INSTR", "timeout (10sec)"=u32 1000, "baud rate (9600)"=u32 38400, "data bits (8)"=u16 8, "parity (0:none)"=enum16{"None", "Odd", "Even", "Mark", "Space"}."None", "stop bits (10: 1 bit)"=w20, "flow control (0:none)"=w21) -> ("VISA resource name out"=w17:refnum<visa-resource-name>, "error out"=w16:errorcluster)  [unwired: 7 in]
  n68 = for {
    tunnel: w98 -> [w246] mode=indexing
    tunnel: [w245] -> w97 mode=indexing
    n69 = property class="Ctl"(reference=w246) -> ("Label.Text"=w245:string)  [unwired: 1 in, 2 out]
  }
  n70 = Divide(x=w73, y=1000000.0) -> (x/y=w72:dbl)
  n71 = Initialize Array(0, 32 ("dimension size")) -> (w5:i32[])
  n72 = Initialize Array(0, 32 ("dimension size")) -> (w1:i32[])
  n73 = VISA Clear(VISA resource name=w17, error in (no error)=w16) -> (VISA resource name out=w15:refnum<visa-resource-name>, error out=w14:errorcluster)
  n74 = Initialize Array(0.0 ("element"), 1 ("dimension size")) -> (w33:dbl[])
  n75 = Initialize Array(0.0 ("element"), 1 ("dimension size")) -> (w30:dbl[])
  n76 = Initialize Array(0.0 ("element"), 1 ("dimension size")) -> (w32:dbl[])
  n77 = Initialize Array(0.0 ("element"), 0 ("dimension size"), 32 ("dimension size")) -> (w31:dbl[][])
  n78 = node-c288(i64 50 ("Period")) -> (w71:T14)  [unwired: 3 in]
  n79 = Initialize Array(0.0 ("element"), 32 ("dimension size")) -> (w27:dbl[])
  n80 = node-c288(w74) -> (w80:T14)  [unwired: 3 in]
  n81 = node-c288(i64 200 ("Period")) -> (w12:T14)  [unwired: 3 in]
  n82 = node-c288(i64 15625 ("Period")) -> (w26:T14)  [unwired: 3 in]
  n83 = node-c288(i64 5 ("Period")) -> (w91:T14)  [unwired: 3 in]
  n84 = node-c288(i64 5 ("Period")) -> (w87:T14)  [unwired: 3 in]
  n85 = while {
    tunnel: w83 -> [w362]
    i -> [w356]
    stop <- w370 stop-if-true
    w261 = 0.0
    w276 = ScalingEnum."Model scale -> Full scale" ("Scale Dir")
    # "Disabled due to resource use"
    # "Manually enter wind speed for now"
    # "Note: This WE is NOT available in the standard version of ROSCO. Need to add in ROSCO src code."
    # "TSR = r * omega / u"
    # "MN x rad/s -> MW"
    # "Note: At e.g. 250ms, a chart history of 500 points equates to 20 of real time"
    # "Display/Graphics Loop (non-RT)"
    n86 = disable-structure shown="Disabled" {
      frame Disabled {
        n87 = shared-variable ".\\SharedVars.lvlib\\RoscoParams"() -> (w375:T13)  [unwired: 1 in, 1 out]
        n88 = Unbundle By Name(w375) -> ("avrSWAP"=→"avrSWAP":dbl[], "aviFAIL"=→"aviFAIL":i32, "currentMsg"=→"Rosco Interface Current Message":string, "firstMsg"=→"Rosco Interface First Message":string)
      }
      frame Enabled {
      }
    }
    n89 = shared-variable ".\\SharedVars.lvlib\\IOSignals"() -> (w248:T11)  [unwired: 1 in, 1 out]
    n90 = shared-variable ".\\SharedVars.lvlib\\PitchAxis1State"() -> (w292:T8)  [unwired: 1 in, 1 out]
    n91 = shared-variable ".\\SharedVars.lvlib\\PitchAxis2State"() -> (w285:T8)  [unwired: 1 in, 1 out]
    n92 = shared-variable ".\\SharedVars.lvlib\\PitchAxis3State"() -> (w278:T8)  [unwired: 1 in, 1 out]
    n93 = shared-variable ".\\SharedVars.lvlib\\GenCtrlFS"() -> (w336:T19)  [unwired: 1 in, 1 out]
    n94 = shared-variable ".\\SharedVars.lvlib\\GenCtrlMS"() -> (w351:T19)  [unwired: 1 in, 1 out]
    n95 = shared-variable ".\\SharedVars.lvlib\\RoscoPairs"() -> (w364:T9)  [unwired: 1 in, 1 out]
    n96 = shared-variable ".\\SharedVars.lvlib\\PitchCtrlMS"() -> (w353:T20)  [unwired: 1 in, 1 out]
    n97 = Tick Count (ms)() -> (millisecond timer value=w363:u32)
    n98 = disable-structure shown="Disabled" {
      frame Disabled {
        # "bytes -> Gb"
        # "TODO - MAKE THIS AND + HOME"
        n99 = Get Volume Info(11:path "C:/" ("path")) -> (2:w381:i64)  [unwired: 1 in, 5 out]
        n100 = To Double Precision Float(number=w381) -> (double precision float=w380:dbl)
        n101 = Divide(x=w380, y=1073741824.0) -> (x/y=w378:dbl)
        "Free GB disk" <- w378
        n102 = Greater?(x=w378, y=2.0) -> (0:→"Disk > 2GB free?":bool)
      }
      frame Enabled {
      }
    }
    n103 = Wait (ms)(milliseconds to wait=u32 250 ("Period")) -> ()  [unwired: 1 out]
    n104 = Subtract(x=w363, y=w362) -> (x-y=w359:u32)
    n105 = disable-structure shown="Disabled" {
      frame Disabled {
        n106 = shared-variable ".\\SharedVars.lvlib\\GeneratorOn"() -> (w393:bool)  [unwired: 1 in, 1 out]
        n107 = shared-variable ".\\SharedVars.lvlib\\PitchAxis1State"() -> (w392:T8)  [unwired: 1 in, 1 out]
        n108 = shared-variable ".\\SharedVars.lvlib\\PitchAxis2State"() -> (w391:T8)  [unwired: 1 in, 1 out]
        n109 = shared-variable ".\\SharedVars.lvlib\\PitchAxis3State"() -> (w390:T8)  [unwired: 1 in, 1 out]
        n110 = case shown="False" w393 {
          frame False {
            n111 = property on="Next Op mode" class="RadioBtnsControl (strict)"("DisabledEnum"=T17."Disabled and Grayed Out" ("Disabled")) -> ()  [unwired: 2 in, 2 out]
            n112 = property on="Enable Accelnet" class="Bool (strict)"("Value"=FALSE ("Enable Accelnet")) -> ()  [unwired: 2 in, 2 out]
            n113 = property on="Next OP mode" class="RadioBtnsControl (strict)"("Value"=GenMode."Velocity: Zero" ("Next OP mode")) -> ()  [unwired: 2 in, 2 out]
          }
          frame True {
            n114 = property on="Next Op mode" class="RadioBtnsControl (strict)"("DisabledEnum"=T17."Enabled" ("Disabled")) -> ()  [unwired: 2 in, 2 out]
          }
        }
        n115 = Unbundle By Name(w392) -> ("Elmo Operational"=w389:bool, "Blade Homed"=w388:bool)
        n116 = Unbundle By Name(w391) -> ("Elmo Operational"=w387:bool, "Blade Homed"=w386:bool)
        n117 = Unbundle By Name(w390) -> ("Elmo Operational"=w385:bool, "Blade Homed"=w384:bool)
        n118 = Compound Arithmetic op=AND(w389, w388, w387, w386, w385, w384) -> (w383:bool)
        n119 = case shown="False" w383 {
          frame False {
            n120 = property on="Next OP mode" class="RadioBtnsControl (strict)"("DisabledEnum"=T17."Disabled and Grayed Out" ("Disabled")) -> ()  [unwired: 2 in, 2 out]
          }
          frame True {
            n121 = property on="Next OP mode" class="RadioBtnsControl (strict)"("DisabledEnum"=T17."Enabled" ("Disabled")) -> ()  [unwired: 2 in, 2 out]
          }
        }
      }
      frame Enabled {
      }
    }
    n122 = To Double Precision Float(number=w356) -> (double precision float=w357:dbl)
    n123 = To Double Precision Float(number=w359) -> (double precision float=w358:dbl)
    n124 = Unbundle By Name(w248) -> ("mainGenVelocity (rad/s)"=w302:dbl)
    n125 = Unbundle By Name(w248) -> ("motorCurrentTorq (Nm)"=w317:dbl, "torqueSensor (Nm)"=w321:dbl)
    "Torque Sensor (Nm) - NOT scaled" <- w321
    "MotorCurrentTorq (Nm)" <- w317
    n126 = shared-variable ".\\SharedVars.lvlib\\GenTorqueSetpoint_Nm"() -> (w320:dbl)  [unwired: 1 in, 1 out]
    n127 = shared-variable ".\\SharedVars.lvlib\\MotorDemandTorque_Nm"() -> (→"MotorDemandTorque_Nm":dbl)  [unwired: 1 in, 1 out]
    n128 = shared-variable ".\\SharedVars.lvlib\\PitchSetpoint_rad"() -> (w354:dbl)  [unwired: 1 in, 1 out]
    n129 = Unbundle By Name(w248) -> ("pitch1Position (rad)"=w340:dbl, "pitch2Position (rad)"=w339:dbl, "pitch3Position (rad)"=w338:dbl)
    n130 = Unbundle By Name(w248) -> ("anemoRefU_m_s"=→"anemoRefU_m_s":dbl)
    n131 = Unbundle By Name(w248) -> ("mainGenVelocity (rad/s)"=w328:dbl)
    n132 = shared-variable ".\\SharedVars.lvlib\\GenVelocitySetpoint_radps"() -> (w329:dbl)  [unwired: 1 in, 1 out]
    n133 = shared-variable ".\\SharedVars.lvlib\\RoscoParams"() -> (w304:T13)  [unwired: 1 in, 1 out]
    n134 = Unbundle By Name(w248) -> ("nacelleAccX (m/s2)"=w252:dbl, "nacelleAccY (m/s2)"=w251:dbl, "nacelleAccZ (m/s2)"=w250:dbl)
    "nacelleAccX (m/s2)" <- w252
    "nacelleAccY (m/s2)" <- w251
    "nacelleAccZ (m/s2)" <- w250
    n135 = Unbundle By Name(w248) -> ("towerTopFx (N)"=w269:dbl, "towerTopFy (N)"=w270:dbl, "towerBotMy (Nm)"=w271:dbl)
    n136 = Unbundle By Name(w364) -> ("BladePitchSetpoint_rad.Value"=→"Rosco Pitch Setpoint (rad)":dbl, "TorqueSetpoint_Nm.Value"=→"Rosco Setpoint (Nm) - MS":dbl, "Out.RotSpeed.Value"=→"OUT_ROTSP":dbl, "OUT_AEROTQ.Value"=→"OUT_AEROTQ":dbl)
    n137 = Divide(x=w358, y=1000.0) -> (x/y=→"Graphics Update t (s)":dbl)
    n138 = Unbundle By Name(w292) -> ("Elmo Operational"=→"Axis 1 Operational":bool, "Elmo Warning"=→"Axis 1 Warning":bool, "Elmo Fault"=→"Axis 1 Fault":bool, "Blade Homing"=→"Axis 1 Homing":bool, "Blade Homed"=→"Axis 1 Homed":bool, "HomePos (rad)"=→"Axis 1 HomePos (rad)":dbl)
    n139 = Unbundle By Name(w285) -> ("Elmo Operational"=→"Axis 2 Operational":bool, "Elmo Warning"=→"Axis 2 Warning":bool, "Elmo Fault"=→"Axis 2 Fault":bool, "Blade Homing"=→"Axis 2 Homing":bool, "Blade Homed"=→"Axis 2 Homed":bool, "HomePos (rad)"=→"Axis 2 HomePos (rad)":dbl)
    n140 = Unbundle By Name(w278) -> ("Elmo Operational"=→"Axis 3 Operational":bool, "Elmo Warning"=→"Axis 3 Warning":bool, "Elmo Fault"=→"Axis 3 Fault":bool, "Blade Homing"=→"Axis 3 Homing":bool, "Blade Homed"=→"Axis 3 Homed":bool, "HomePos (rad)"=→"Axis 3 HomePos (rad)":dbl)
    n141 = Unbundle By Name(w336) -> ("Constant velocity setpoint (rpm)"=→"Const. vel setpoint FS (rpm)":dbl, "Ramp target velocity (rpm)"=→"Ramp target vel FS (rpm)":dbl, "Ramp time (s)"=→"Ramp time FS (s)":dbl, "Sine mean (Nm)"=→"Torque sine mean FS (Nm)":dbl, "Sine amp (Nm)"=→"Torque sine amp FS (Nm)":dbl, "Sine period (s)"=→"Torque sine period FS (Nm)":dbl)
    n142 = Divide(x=w358, y=w357) -> (x/y=→"Effective graphics rate (ms)":dbl)
    n143 = Unbundle By Name(w351) -> ("Generator operating mode"=→"Current OP mode":T2, "Constant velocity setpoint (rpm)"=→"Const. vel setpoint MS (rpm)":dbl, "Ramp target velocity (rpm)"=→"Ramp target vel MS (rpm)":dbl, "Ramp time (s)"=→"Ramp time MS (s)":dbl, "Sine mean (Nm)"=→"Torque sine mean MS (Nm)":dbl, "Sine amp (Nm)"=→"Torque sine amp MS (Nm)":dbl, "Sine period (s)"=→"Torque sine period MS (Nm)":dbl)
    n144 = Unbundle By Name(w353) -> ("Constant setpoint (deg)"=→"Current Const. (deg)":dbl, "Blade pitch operating mode"=→"Current OP mode":T4)
    n145 = shared-variable ".\\SharedVars.lvlib\\Const"() -> (w307:T1)  [unwired: 1 in, 1 out]
    n146 = Unbundle By Name(w304) -> ("avrSWAP"=w301:dbl[])
    n147 = Unbundle By Name(w307) -> ("rotorRadius"=w306:sgl, "scaleFactor"=w273:dbl)
    n148 = case shown="\"Gauges & Scopes Model Scale\"" "IndicatorScale" {
      tunnel: w329 -> [w452 w457]
      tunnel: w328 -> [w453 w458]
      tunnel: [w451 w458] -> w313
      tunnel: [w450 w457] -> w326
      frame "Gauges & Scopes Full Scale", Default {
        w456 = ScalingEnum."Model scale -> Full scale" ("Scale Dir")
        n149 = shared-variable ".\\SharedVars.lvlib\\Const"() -> (w455:T1)  [unwired: 1 in, 1 out]
        n150 = Unbundle By Name(w455) -> ("scaleFactor"=w454:dbl)
        n151 = call "ScaleRotVel.vi"("Scale Dir"=w456, "Scale factor"=w454, "Rotational Velocity (In)"=w452) -> ("Rotational Velocity (Out)"=w450:dbl)  [unwired: 8 in]
        n152 = call "ScaleRotVel.vi"("Scale Dir"=w456, "Scale factor"=w454, "Rotational Velocity (In)"=w453) -> ("Rotational Velocity (Out)"=w451:dbl)  [unwired: 8 in]
      }
      frame "Gauges & Scopes Model Scale" {
      }
    }
    n153 = call "RadToDeg.vi"("rad"=w340) -> ("deg"=w325:dbl)
    "Pitch Blade 1 (deg)" <- w325
    n154 = call "RadToDeg.vi"("rad"=w339) -> ("deg"=w324:dbl)
    "Pitch Bade 2 (deg)" <- w324
    n155 = call "RadToDeg.vi"("rad"=w338) -> ("deg"=w323:dbl)
    "Pitch Blade 3 (deg)" <- w323
    n156 = call "RadToDeg.vi"("rad"=w354) -> ("deg"=w343:dbl)
    "Pitch Setpoint (deg)" <- w343
    n157 = Index Array(array=w301, index=199) -> (element=→"WE ROSCO":dbl)
    n158 = Merge Signals(w343, w325, w324, w323) -> (→"Pitch":dynamicdata)
    n159 = Merge Signals(w252, w251, w250) -> (→"Accel":dynamicdata)
    n160 = feedback #1(w261) -> (w254:dbl)
    "FyMean" <- w254
    n161 = feedback #2(w261) -> (w255:dbl)
    "MyMean" <- w255
    n162 = feedback #3(w261) -> (w260:dbl)
    "FxMean" <- w260
    n163 = case shown="True" "Sample" {
      selector: "Sample" -> [_ w425]
      tunnel: w271 -> [w415 w420]
      tunnel: w270 -> [w416 w419]
      tunnel: w269 -> [w417 w418]
      tunnel: [w417 w418] -> w267
      tunnel: [w416 w419] -> w266
      tunnel: [w415 w420] -> w265
      tunnel: [w413 w422] -> w263
      tunnel: [w414 w421] -> w264
      tunnel: [w412 w423] -> w262
      tunnel: w260 -> [w414 _]
      tunnel: w254 -> [w413 _]
      tunnel: w255 -> [w412 _]
      frame False {
      }
      frame True {
        w424 = 100 ("sample length")
        n164 = call <vilib>:"Mean PtByPt.vi"("x"=w418, "sample length"=w424, "initialize"=w425) -> ("mean"=w421:dbl)  [unwired: 1 in, 1 out]
        n165 = call <vilib>:"Mean PtByPt.vi"("x"=w419, "sample length"=w424, "initialize"=w425) -> ("mean"=w422:dbl)  [unwired: 1 in, 1 out]
        n166 = call <vilib>:"Mean PtByPt.vi"("x"=w420, "sample length"=w424, "initialize"=w425) -> ("mean"=w423:dbl)  [unwired: 1 in, 1 out]
      }
    }
    n167 = feedback-in #1(w263) -> ()
    n168 = feedback-in #2(w262) -> ()
    n169 = feedback-in #3(w264) -> ()
    n170 = To Double Precision Float(number=w306) -> (double precision float=w310:dbl)
    n171 = call "ScaleRotVel.vi"("Scale Dir"=w276, "Scale factor"=w273, "Rotational Velocity (In)"=w302) -> ("Rotational Velocity (Out)"=w300:dbl)  [unwired: 8 in]
    n172 = call "ScaleTime.vi"("Scale Dir"=w276, "Scale factor"=w273, "Time (In)"="windSpeed_m_s") -> ("Time OUT (Out)"=w274:dbl)  [unwired: 8 in]
    n173 = case shown="False" "Apply Ofst" {
      tunnel: w267 -> [w402 w411]
      tunnel: w266 -> [w401 w410]
      tunnel: w265 -> [w400 w409]
      tunnel: w260 -> [_ w408]
      tunnel: w254 -> [_ w407]
      tunnel: w255 -> [_ w406]
      tunnel: [w402 w405] -> w259
      tunnel: [w401 w404] -> w258
      tunnel: [w400 w403] -> w257
      frame False {
      }
      frame True {
        n174 = Subtract(x=w410, y=w407) -> (x-y=w404:dbl)
        n175 = Subtract(x=w411, y=w408) -> (x-y=w405:dbl)
        n176 = Subtract(x=w409, y=w406) -> (x-y=w403:dbl)
      }
    }
    n177 = Multiply(x=w310, y=w300) -> (x*y=w309:dbl)
    n178 = Divide(x=w309, y=w274) -> (x/y=w308:dbl)
    n179 = Merge Signals(w308) -> ()  [unwired: 1 out]
    n180 = case shown="\"Gauges & Scopes Model Scale\"" "IndicatorScale" {
      tunnel: w321 -> [w438 w449]
      tunnel: [w443 w449] -> w314
      tunnel: w320 -> [w437 w448]
      tunnel: [w442 w448] -> w315
      tunnel: w317 -> [w436 w447]
      tunnel: [w434 w447] -> w316
      tunnel: [w433 w446] -> w277
      tunnel: [w432 w445] -> w256
      tunnel: [w430 w444] -> w253
      tunnel: w259 -> [w428 w446]
      tunnel: w258 -> [w427 w445]
      tunnel: w257 -> [w426 w444]
      frame "Gauges & Scopes Full Scale", Default {
        w431 = ScalingEnum."Model scale -> Full scale" ("Scale Dir")
        n181 = shared-variable ".\\SharedVars.lvlib\\Const"() -> (w439:T1)  [unwired: 1 in, 1 out]
        n182 = Unbundle By Name(w439) -> ("scaleFactor"=w429:dbl)
        n183 = call "ScaleTorque.vi"("Scale Dir"=w431, "Scale factor"=w429, "Torque (In)"=w436) -> ("Torque (Out)"=w435:dbl)  [unwired: 8 in]
        n184 = call "ScaleTorque.vi"("Scale Dir"=w431, "Scale factor"=w429, "Torque (In)"=w438) -> ("Torque (Out)"=w441:dbl)  [unwired: 8 in]
        n185 = call "ScaleTorque.vi"("Scale Dir"=w431, "Scale factor"=w429, "Torque (In)"=w437) -> ("Torque (Out)"=w440:dbl)  [unwired: 8 in]
        n186 = call "ScaleTorque.vi"("Scale Dir"=w431, "Scale factor"=w429, "Torque (In)"=w426) -> ("Torque (Out)"=w430:dbl)  [unwired: 8 in]
        n187 = call "ScaleForce.vi"("Scale Dir"=w431, "Scale factor"=w429, "Force (In)"=w428) -> ("Force (Out)"=w433:dbl)  [unwired: 8 in]
        n188 = call "ScaleForce.vi"("Scale Dir"=w431, "Scale factor"=w429, "Force (In)"=w427) -> ("Force (Out)"=w432:dbl)  [unwired: 8 in]
        n189 = call "NumBy1E6.vi"("x"=w435) -> ("Mx"=w434:dbl)
        n190 = call "NumBy1E6.vi"("x"=w441) -> ("Mx"=w443:dbl)
        n191 = call "NumBy1E6.vi"("x"=w440) -> ("Mx"=w442:dbl)
      }
      frame "Gauges & Scopes Model Scale" {
      }
    }
    "Torque Setpoint" <- w315
    "Torque Cell" <- w314
    "Fx" <- w277
    "Fy" <- w256
    "towerBotMy" <- w253
    n192 = call "RadpsToRPM.vi"("radps"=w313) -> ("rpm"=w342:dbl)
    "Actual Speed MS (rpm)" <- w342
    n193 = call "RadpsToRPM.vi"("radps"=w326) -> ("rpm"=w327:dbl)
    "Speed Setpoint (rpm)" <- w327
    n194 = Compound Arithmetic op=MULTIPLY(w313, w314) -> (→"Power (MW)":dbl)
    n195 = Merge Signals(w327, w342) -> (w341:dynamicdata)
    n196 = Merge Signals(w341) -> (→"Generator Speed":dynamicdata)
    n197 = shared-variable ".\\SharedVars.lvlib\\StopLabVIEW"() -> (w370:bool)  [unwired: 1 in, 1 out]
    n198 = Merge Signals(w315, w314, w316, w277, w256, w253) -> (→"Rotor Loads":dynamicdata)
  }
  n199 = timed-loop {
    timing: w71 -> [_]
    timing-out: [_] -> w70
    shift-right: [w537] -> _
    shift-left: BladePitchMode."Zero pitch" ("PitchCtrlMode") -> [w554]
    shift-right: [w538] -> _
    shift-left: 0.0 -> [w552]
    shift-right: [w497] -> _
    shift-left: GenMode."Velocity: Zero" ("GenOpMode") -> [w550]
    shift-right: [w513] -> _
    shift-left: 0.0 -> [w523]
    shift-right: [w511] -> _
    shift-left: 5.0 -> [w522]
    shift-right: [w510] -> _
    shift-left: 100.0 -> [w521]
    shift-right: [w506] -> _
    shift-left: 0.0 -> [w520]
    shift-right: [w505] -> _
    shift-left: 0.0 -> [w519]
    shift-right: [w504] -> _
    shift-left: 0.0 -> [w518]
    shift-right: [w482] -> _
    shift-left: w33 -> [w487]
    shift-right: [w478] -> _
    shift-left: w30 -> [w486]
    shift-right: [w477] -> _
    shift-left: w32 -> [w485]
    shift-right: [w468] -> _
    shift-left: w31 -> [w484]
    shift-right: [w464] -> _
    shift-left: w27 -> [w465]
    stop <- w561 stop-if-true
    w508 = 1000000.0 ("y")
    w536 = T19 {"Constant velocity setpoint (rpm)"=0.0, "Ramp target velocity (rpm)"=0.0, "Ramp time (s)"=0.0, "Sine mean (Nm)"=0.0, "Sine amp (Nm)"=0.0, "Sine period (s)"=0.0, "Torque Ctrl I-Gain"=0.0, "Velocity Ctrl P-Gain"=0.0, "Velocity Ctrl I-Gain"=0.0, "Max Torque (Nm)"=0.0, "GeneratorOn"=FALSE, "Torque Ctrl P-Gain"=0.0, "From file velocity (rpm)"=0.0, "Generator operating mode"=enum."Velocity: Zero", "Max Vel (rpm)"=0.0, "Torque Ctrl FF Gain"=0.0}  # Gen Control
    w541 = T20 {"P-Gain"=0.0, "Blade pitch operating mode"=enum."From File", "Constant setpoint (deg)"=0.0, "I-Gain"=0.0, "Pitch from File (deg)"=0.0, "Homing vel (rpm)"=0.0, "Max vel (rpm)"=0.0, "Max vel change (rpm/min)"=0.0}  # PitchCtrl
    # "Probably not required, but leave in cluster if needed"
    # "This code finds the NEAREST LOWER time. For example, if elements 40s and 50s exist in the input time vector, and tnow = 49s, the code will find the index for 40s."
    # "MNm-> Nm"
    # "Scale right after user input"
    # "Scale right after user input"
    # "MNm-> Nm"
    # "File setpoint and mode loop (RT, but only at 50 ms)"
    n200 = node-c288() -> (→"Loop duration (ms)":i64)  [unwired: 1 in]
    n201 = First Call?() -> (First Call?: T/F=w459:bool)
    n202 = Or(x=w459, y="Reload File") -> (x .or. y?=w461:bool)
    n203 = case shown="True" w461 {
      tunnel: "Setpoint file name" -> [_ w600]
      tunnel: [w592 w597] -> w482
      tunnel: [w590 w596] -> w478
      tunnel: [w589 w595] -> w477
      tunnel: [w591 w594] -> w468
      tunnel: w487 -> [w592 _]
      tunnel: w486 -> [w590 _]
      tunnel: w485 -> [w589 _]
      tunnel: w484 -> [w591 _]
      frame False {
      }
      frame True {
        n204 = call "ReadSetpointFile-v2.vi"("Setpoint file name"=w600) -> ("Fan Vel Set"=w594:dbl[][], "Rotor Spd Set"=w595:dbl[], "Pitch Set"=w596:dbl[], "Time"=w597:dbl[], "Setpoint file loaded"=→"Setpoint file loaded":path, "Setpoint indicator"=→"Setpoints":dbl[][], "Read error"=→"Setpoint read error":string)  [unwired: 4 in]
      }
    }
    n205 = shared-variable ".\\SharedVars.lvlib\\ExpTime_s"() -> (w560:dbl)  [unwired: 1 in, 1 out]
    n206 = shared-variable ".\\SharedVars.lvlib\\Const"() -> (w559:T1)  [unwired: 1 in, 1 out]
    n207 = case shown="True" "Commit" {
      tunnel: "Fan Setpoint (%)" -> [_ w606]
      tunnel: w465 -> [w601 _]
      tunnel: [w601 w602] -> w464
      frame False {
      }
      frame True {
        n208 = Initialize Array(1.0 ("element"), 32 ("dimension size")) -> (w603:dbl[])
        n209 = Multiply(x=w606, y=w603) -> (x*y=w602:dbl[])
      }
    }
    n210 = case shown="True" "Commit gen settings" {
      tunnel: w550 -> [w570 _]
      tunnel: [w570 w577] -> w496
      tunnel: "Next OP mode" -> [_ w577]
      tunnel: "Const. vel (rpm)" -> [_ w576]
      tunnel: "Ramp target vel (rpm)" -> [_ w575]
      tunnel: "Ramp time (s)" -> [_ w574]
      tunnel: "Torque mean (MNm)" -> [_ w573]
      tunnel: "Torque sine amp (MNm)" -> [_ w572]
      tunnel: "Torque sine period (s)" -> [_ w571]
      tunnel: w523 -> [w569 _]
      tunnel: w522 -> [w568 _]
      tunnel: w521 -> [w567 _]
      tunnel: w520 -> [w566 _]
      tunnel: w519 -> [w565 _]
      tunnel: w518 -> [w564 _]
      tunnel: [w569 w576] -> w513
      tunnel: [w568 w575] -> w511
      tunnel: [w567 w574] -> w510
      tunnel: [w566 w573] -> w506
      tunnel: [w565 w572] -> w505
      tunnel: [w564 w571] -> w504
      frame False {
      }
      frame True {
      }
    }
    n211 = shared-variable ".\\SharedVars.lvlib\\GeneratorOn"() -> (w498:bool)  [unwired: 1 in, 1 out]
    n212 = Unbundle By Name(w559) -> ("scaleFactor"=w558:dbl)
    n213 = case shown="True" "Commit pitch settings" {
      tunnel: w554 -> [w617 _]
      tunnel: [w617 w619] -> w537
      tunnel: "Next OP mode" -> [_ w619]
      tunnel: w552 -> [w616 _]
      tunnel: [w616 w618] -> w538
      tunnel: "Next Const. (deg)" -> [_ w618]
      frame False {
      }
      frame True {
      }
    }
    n214 = call "ScaleTime.vi"("Scale Dir"=ScalingEnum."Model scale -> Full scale", "Scale factor"=w558, "Time (In)"=w560) -> ("Time OUT (Out)"=w556:dbl)  [unwired: 8 in]
    "Exp time FS (s)" <- w556
    n215 = case shown="False" w498 {
      tunnel: [GenMode."Velocity: Zero" ("Next OP mode") w563] -> w497
      tunnel: w496 -> [_ w563]
      frame False {
      }
      frame True {
      }
    }
    n216 = Subtract(x=w482, y=w556) -> (x-y=w483:dbl[])
    n217 = shared-variable ".\\SharedVars.lvlib\\FromFileVelFS_rpm"() -> (w530:dbl)  [unwired: 1 in, 1 out]
    n218 = shared-variable ".\\SharedVars.lvlib\\GeneratorOn"() -> (w528:bool)  [unwired: 1 in, 1 out]
    n219 = shared-variable ".\\SharedVars.lvlib\\FromFilePitchFS_deg"() -> (w539:dbl)  [unwired: 1 in, 1 out]
    n220 = Array Size(array=w483) -> (size(s)=w500:i32)
    n221 = Less Or Equal To 0?(x=w483) -> (x <= 0?=w501:bool[])
    n222 = for {
      N: w500 -> [_]
      tunnel: w501 -> [w610] mode=indexing
      shift-right: [w607] -> w481
      shift-left: w483 -> [w609]
      i -> [w608]
      n223 = case shown="False" w610 {
        tunnel: w609 -> [w611 w615]
        tunnel: w608 -> [w614 _]
        tunnel: [w612 w615] -> w607
        frame False {
          n224 = Replace Array Subset(array=w611, new element=nan ("new element/subarray"), index=w614) -> (w612:dbl[])
        }
        frame True {
        }
      }
    }
    n225 = Multiply(x=1000000.0 ("y"), y="Max Torque (MNm) - FS") -> (x*y=w534:dbl)
    n226 = Multiply(x=w508, y=w506) -> (x*y=w509:dbl)
    n227 = Multiply(x=w505, y=w508) -> (x*y=w507:dbl)
    n228 = shared-variable ".\\SharedVars.lvlib\\Const"() -> (w494:T1)  [unwired: 1 in, 1 out]
    n229 = shared-variable ".\\SharedVars.lvlib\\Const"() -> (w527:T1)  [unwired: 1 in, 1 out]
    n230 = Bundle By Name(cluster=w541, "Blade pitch operating mode"=w537, "P-Gain"="Pitch P-Gain", "I-Gain"=0.0, "Constant setpoint (deg)"=w538, "Pitch from File (deg)"=w539, "Homing vel (rpm)"="Pitch Homing Vel  (rpm) - FS", "Max vel (rpm)"="Pitch Max Vel (rpm) - FS", "Max vel change (rpm/min)"="Pitch Max Vel Change (rpm/min) - FS") -> (w514:T20)
    n231 = Bundle By Name(cluster=w536, "Sine period (s)"=w504, "Sine amp (Nm)"=w507, "Sine mean (Nm)"=w509, "Ramp time (s)"=w510, "Ramp target velocity (rpm)"=w511, "Constant velocity setpoint (rpm)"=w513, "Generator operating mode"=w497, "GeneratorOn"=w528, "From file velocity (rpm)"=w530, "Max Torque (Nm)"=w534, "Max Vel (rpm)"="Max Vel (rpm)  -FS", "Torque Ctrl P-Gain"="Torque Ctrl P-Gain", "Torque Ctrl I-Gain"="Torque Ctrl I-Gain", "Torque Ctrl FF Gain"="Torque Ctrl FF Gain", "Velocity Ctrl P-Gain"="Velocity Ctrl P-Gain", "Velocity Ctrl I-Gain"="Velocity Ctrl I-Gain") -> (w512:T19)
    n232 = Absolute Value(x=w481) -> (abs(x)=w480:dbl[])
    n233 = Unbundle By Name(w494) -> ("scaleFactor"=w515:dbl)
    n234 = Array Max & Min(array=w480) -> (min index (indices)=w466:i32)  [unwired: 3 out]
    "Time index" <- w466
    n235 = Array Subset(array=w468, index (row)=w466, length (row)=1 ("length")) -> (w467:dbl[][])  [unwired: 2 in]
    n236 = Reshape Array(w467, 32 ("dimension size")) -> (w475:dbl[])
    n237 = case shown="\"Manual\", Default" "Ctrl Mode" {
      tunnel: [TRUE ("ManualOn") FALSE ("ManualOn")] -> _
      tunnel: [FALSE ("ManualOn") TRUE ("ManualOn")] -> _
      tunnel: [w581 w586] -> w471
      tunnel: w475 -> [_ w586]
      tunnel: w464 -> [w582 _]
      frame "Manual", Default {
        # "From % to [0,1]"
        n238 = Divide(x=w582, y=100.0) -> (x/y=w581:dbl[])
      }
      frame "FromFile" {
      }
    }
    n239 = Unbundle By Name(w527) -> ("scaleFactor"=w526:dbl)
    n240 = In Range and Coerce(upper limit=1.0, x=w471, lower limit=0.0) -> (coerced(x)=w463:dbl[])  [unwired: 1 out]
    "Current Setting" <- w463
    n241 = call "ScalePitchCtrl.vi"("Scale Direction"=ScalingEnum."Full scale -> Model scale", "Scale Factor"=w515, "PitchCtrl (In)"=w514) -> ("PitchCtrl (Out)"=w517:T20)  [unwired: 8 in]
    n242 = Index Array(array=w478, index=w466) -> (element=w474:dbl)
    "From File Pitch FS (deg)" <- w474
    n243 = Index Array(array=w477, index=w466) -> (element=w462:dbl)
    "From File RotSpd FS (rpm)" <- w462
    n244 = shared-variable ".\\SharedVars.lvlib\\StopLabVIEW"() -> (w561:bool)  [unwired: 1 in, 1 out]
    n245 = call "ScaleGenCtrl.vi"("Scale Dir"=ScalingEnum."Full scale -> Model scale", "Scale factor"=w526, "Gen Control (In)"=w512) -> ("Gen Control (Out)"=w524:T19)  [unwired: 8 in]
    n246 = shared-variable ".\\SharedVars.lvlib\\PitchCtrlFS"(w514) -> ()  [unwired: 1 in, 1 out]
    n247 = shared-variable ".\\SharedVars.lvlib\\FromFilePitchFS_deg"(w474) -> ()  [unwired: 1 in, 1 out]
    n248 = shared-variable ".\\SharedVars.lvlib\\FromFileVelFS_rpm"(w462) -> ()  [unwired: 1 in, 1 out]
    n249 = shared-variable ".\\SharedVars.lvlib\\FanSetpoint_unit"(w463) -> ()  [unwired: 1 in, 1 out]
    n250 = shared-variable ".\\SharedVars.lvlib\\PitchCtrlMS"(w517) -> ()  [unwired: 1 in, 1 out]
    n251 = shared-variable ".\\SharedVars.lvlib\\GenCtrlFS"(w512) -> ()  [unwired: 1 in, 1 out]
    n252 = shared-variable ".\\SharedVars.lvlib\\GenCtrlMS"(w524) -> ()  [unwired: 1 in, 1 out]
    n253 = node-c288() -> ()  [unwired: 1 in, 1 out]
  }
  n254 = timed-loop {
    timing: w80 -> [_]
    timing-out: [_] -> w79
    shift-right: [w622] -> _
    shift-left: w92 -> [w663]
    shift-right: [w623] -> w77
    shift-left: errorcluster {"status"=FALSE, "code"=0, "source"=""} ("error out") -> [w662]
    shift-right: [w637] -> _
    shift-left: T9 {"iStatus"={"Index"=0, "Value"=0.0}, "TIME"={"Index"=1, "Value"=0.0}, "DT"={"Index"=2, "Value"=0.0}, "Blade1PitchPos_rad"={"Index"=3, "Value"=0.0}, "VS_MECHGENPWR"={"Index"=13, "Value"=0.0}, "VS_GENPWR"={"Index"=14, "Value"=0.0}, "GEN_SPEED"={"Index"=19, "Value"=0.0}, "ROTOR_SPEED"={"Index"=20, "Value"=0.0}, "GENTQMEAS"={"Index"=22, "Value"=0.0}, "Y_M"={"Index"=23, "Value"=0.0}, "HORWINDV"={"Index"=26, "Value"=0.0}, "ROOTMOOP1"={"Index"=29, "Value"=0.0}, "ROOTMOOP2"={"Index"=30, "Value"=0.0}, "Blade2PitchPos_rad"={"Index"=32, "Value"=0.0}, "Blade3PitchPos_rad"={"Index"=33, "Value"=0.0}, "ROOTMOOP3"={"Index"=31, "Value"=0.0}, "AVCMSG_SIZE"={"Index"=48, "Value"=0.0}, "INFILE_SIZE "={"Index"=49, "Value"=0.0}, "OUTFILE_SIZE "={"Index"=50, "Value"=0.0}, "FA_ACC"={"Index"=52, "Value"=0.0}, "NUM_BLADES"={"Index"=60, "Value"=0.0}, "BladePitchSetpoint_rad"={"Index"=44, "Value"=0.0}, "TorqueSetpoint_Nm"={"Index"=46, "Value"=0.0}, "OUT_AEROTQ"={"Index"=91, "Value"=0.0}, "Out.RotSpeed "={"Index"=92, "Value"=0.0}, "Out.DEBUG"={"Index"=93, "Value"=0.0}} ("ArrayPairs") -> [w664]
    shift-right: [w633] -> _
    shift-left: T11 {"mainGenPosition (rad)"=0.0, "motorCurrentTorq (Nm)"=0.0, "mainGenVelocity (rad/s)"=0.0, "mainGenStatus"=0, "pitch1Position (rad)"=0.0, "pitch1Velocity (rad/s)"=0.0, "pitch1Status"=0, "pitch2Position (rad)"=0.0, "pitch2Velocity (rad/s)"=0.0, "pitch2Status"=0, "pitch3Position (rad)"=0.0, "pitch3Velocity (rad/s)"=0.0, "pitch3Status"=0, "torqueSensor (Nm)"=0.0, "nacelleAccX (m/s2)"=0.0, "nacelleAccY (m/s2)"=0.0, "nacelleAccZ (m/s2)"=0.0, "pitch1HomeFlag"=FALSE, "pitch2HomeFlag"=FALSE, "pitch3HomeFlag"=FALSE, "towerTopFx (N)"=0.0, "towerTopFy (N)"=0.0, "towerBotMy (Nm)"=0.0, "anemoRefU_m_s"=0.0, "anemoRefV_m_s"=0.0, "anemoRefW_m_s"=0.0} -> [w661]
    tunnel: w72 -> [w658]
    tunnel: w72 -> [w657]
    i -> [w624]
    stop <- w667 stop-if-true
    # "Main/Control/Execution Loop"
    n255 = node-c288() -> (→"RT Loop Late?":bool, →"RT Loop Duration":i64)  [unwired: 1 in]
    n256 = shared-variable ".\\SharedVars.lvlib\\AnemometerData"() -> ()  [unwired: 1 in, 2 out]
    n257 = shared-variable ".\\SharedVars.lvlib\\PitchAxis3State"() -> (w625:T8)  [unwired: 1 in, 1 out]
    n258 = shared-variable ".\\SharedVars.lvlib\\PitchAxis2State"() -> (w626:T8)  [unwired: 1 in, 1 out]
    n259 = shared-variable ".\\SharedVars.lvlib\\PitchAxis1State"() -> (w627:T8)  [unwired: 1 in, 1 out]
    n260 = To Double Precision Float(number=w624) -> (double precision float=w659:dbl)
    n261 = call "ReadIO.vi"("ArrayPairs In"=w664, "PitchAxis1State"=w627, "PitchAxis2State"=w626, "PitchAxis3State"=w625, "IO Signals In"=w661, "ROSCO Params In"=w663, "error in"=w662) -> ("ArrayPairs Out"=w656:T9, "IO Signals Out"=w653:T11, "ROSCO Params Out"=w655:T13, "Torque RAW (V)"=→"Torque RAW (V)":dbl, "error out"=w654:errorcluster)  [unwired: 4 in]
    n262 = Multiply(x=w659, y=w658) -> (x*y=w632:dbl)
    "cRio Time(s)" <- w632
    n263 = call "AssignStatus_v2.vi"("Time (s)"=w632, "Rosco dt (s)"=w657, "LoopCount"=w624, "Wind Estimator u(t=0) FS"="Wind Est. u(t=0)", "error in (no error)"=w654, "ROSCO Params In"=w655, "IO Signals In"=w653, "ArrayPairs In"=w656) -> ("error out"=w650:errorcluster, "ROSCO Params Out"=w651:T13, "IO Signals Out"=w649:T11, "ArrayPairs Out"=w652:T9)
    n264 = shared-variable ".\\SharedVars.lvlib\\CtrlLoopTime_s"(w632) -> ()  [unwired: 1 in, 1 out]
    n265 = call "CreateSwapArray_v4.vi"("Loop count"=w624, "error in (no error)"=w650, "ROSCO Params"=w651, "IO Signals In"=w649, "ArrayPairs"=w652) -> ("error out"=w645:errorcluster, "ROSCO Params Out"=w646:T13, "IO Signals Out"=w644:T11, "ArrayPairs Out"=w647:T9)  [unwired: 3 in]
    n266 = shared-variable ".\\SharedVars.lvlib\\PitchCtrlMS"() -> (w631:T20)  [unwired: 1 in, 1 out]
    n267 = call "CallRosco_v2.vi"("StopLV"="Stop LabVIEW", "error in (no error)"=w645, "ROSCO Params in"=w646, "IO Signals In"=w644, "ArrayPairs"=w647) -> ("error out"=w643:errorcluster, "ROSCO Params Out"=w628:T13, "IO Signals Out"=w660:T11, "ArrayPairs Out"=w629:T9)  [unwired: 3 in]
    n268 = call "PitchCtrl.vi"("ArrayPairs In"=w629, "IO Signals In"=w660, "ROSCO Params in"=w628, "error in (no error)"=w643, "PitchCtrl"=w631, "Time (s)"=w632, "PitchAxis1State"=w627, "PitchAxis2State"=w626, "PitchAxis3State"=w625) -> ("Pitch setpoint (rad)"=w642:dbl, "ArrayPairs Out"=w641:T9, "IO Signals Out"=w640:T11, "ROSCO Params Out"=w639:T13, "error out"=w638:errorcluster)  [unwired: 6 in]
    n269 = shared-variable ".\\SharedVars.lvlib\\PitchSetpoint_rad"(w642) -> ()  [unwired: 1 in, 1 out]
    n270 = shared-variable ".\\SharedVars.lvlib\\GenCtrlMS"() -> (w630:T19)  [unwired: 1 in, 1 out]
    n271 = call "GenCtrlCsv.vi"("Loop Time (s)"=w632, "Gen Control"=w630, "error in (no error)"=w638, "ROSCO Params in"=w639, "IO Signals In"=w640, "ArrayPairs In"=w641) -> ("error out"=w623:errorcluster, "ROSCO Params Out"=w622:T13, "IO Signals Out"=w633:T11, "ArrayPairs Out"=w637:T9, "Velocity setpoint (rad/s)"=w634:dbl, "Torque setpoint (Nm)"=w635:dbl)
    n272 = shared-variable ".\\SharedVars.lvlib\\GenTorqueSetpoint_Nm"(w635) -> ()  [unwired: 1 in, 1 out]
    n273 = shared-variable ".\\SharedVars.lvlib\\GenVelocitySetpoint_radps"(w634) -> ()  [unwired: 1 in, 1 out]
    n274 = Unbundle By Name(w622) -> ("aviFAIL"=w620:i32)
    n275 = disable-structure shown="Disabled" {
      disable-tunnel: w622 -> [w669 _]
      frame Disabled {
        n276 = shared-variable ".\\SharedVars.lvlib\\RoscoParams"(w669) -> ()  [unwired: 1 in, 1 out]
      }
      frame Enabled {
      }
    }
    n277 = shared-variable ".\\SharedVars.lvlib\\RoscoPairs"(w637) -> ()  [unwired: 1 in, 1 out]
    n278 = Or(x=w623, y="Stop LabVIEW") -> (x .or. y?=w667:bool)
    n279 = shared-variable ".\\SharedVars.lvlib\\IOSignals"(w633) -> ()  [unwired: 1 in, 1 out]
    n280 = Not Equal To 0?(x=w620) -> (x != 0?=→"Rosco Failed?":bool)
    n281 = shared-variable ".\\SharedVars.lvlib\\StopLabVIEW"(w667) -> ()  [unwired: 1 in, 1 out]
    n282 = node-c288() -> ()  [unwired: 1 in, 1 out]
  }
  n283 = timed-loop {
    timing: w12 -> [_]
    timing-out: [_] -> w11
    shift-right: [w698] -> _
    shift-left: w10 -> [w700]
    shift-right: [w680] -> _
    shift-left: w5 -> [w693]
    shift-right: [w679] -> _
    shift-left: w2 -> [w692]
    shift-right: [w674] -> _
    shift-left: w1 -> [w691]
    shift-right: [w699] -> _
    shift-left: w8 -> [w702]
    stop <- w696 stop-if-true
    w697 = "192.168.1.52"  # PLC IP address
    # "192.168.1.52"
    # "Loop to update the PLC read / write tags"
    n284 = node-c288() -> (→"PLC read/write late?":bool)  [unwired: 1 in]
    n285 = shared-variable ".\\SharedVars.lvlib\\FanSetpoint_unit"() -> (w678:dbl[])  [unwired: 1 in, 1 out]
    n286 = call "ReadPLC.vi"("PLC Current State In"=w700, "PLC IP address"=w697, "PLC Current VFD In"=w693, "PLC Setpoint State In"=w692, "PLC Setpoint VFD In"=w691, "Error In"=w702) -> ("PLC Current State Out"=w690:T7, "PLC Current VFD Out"=w689:i32[], "PLC Setpoint State Out"=w688:T7, "PLC Setpoint VFD Out"=w687:i32[], "Read Error"=→"PLC Read Error":bool, "Read errors"=→"PLC read errors":string, "Error Out"=w686:errorcluster)  [unwired: 3 in]
    n287 = call "PLCCtrl.vi"("PLC Current State In"=w690, "FanSetpoint_uint"=w678, "PLC Current VFD In"=w689, "PLC Setpoint State In"=w688, "PLC Setpoint VFD In"=w687, "Error In"=w686, "Enable Fans"="Enable Fans", "Turn Fans On"="Turn Fans On", "Clear Faults"="Clear Faults") -> ("PLC Current State Out"=w685:T7, "PLC Current VFD Out"=w684:i32[], "PLC Setpoint State Out"=w683:T7, "PLC Setpoint VFD Out"=w682:i32[], "Error Out"=w681:errorcluster)  [unwired: 2 in]
    n288 = call "WritePLC.vi"("PLC Current State In"=w685, "PLC IP address"=w697, "PLC Current VFD In"=w684, "Ctrl Setpoint State In"=w683, "PLC Setpoint VFD In"=w682, "Error In"=w681) -> ("PLC Current State Out"=w698:T7, "PLC Current VFD Out"=w680:i32[], "PLC Setpoint State Out"=w679:T7, "PLC Setpoint VFD Out"=w674:i32[], "Error Out"=w699:errorcluster)  [unwired: 5 in]
    n289 = shared-variable ".\\SharedVars.lvlib\\StopLabVIEW"() -> (w696:bool)  [unwired: 1 in, 1 out]
    n290 = node-c288() -> ()  [unwired: 1 in, 1 out]
  }
  n291 = timed-loop {
    timing: w26 -> [_]
    timing-out: [_] -> w25
    tunnel: w15 -> [w715]
    tunnel: [w715] -> _
    shift-right: [w708] -> _
    shift-left: w14 -> [w714]
    stop <- w711 stop-if-true
    # "22 is a full read for 3 channels and EOL /r"
    # "Loop to update the wind data via RS232"
    n292 = node-c288() -> (→"RS232 loop late?":bool)  [unwired: 1 in]
    n293 = VISA Read(VISA resource name=w715, byte count=u32 22, error in (no error)=w714) -> (VISA resource name out=w710:refnum<visa-resource-name>, read buffer=w707:string, error out=w709:errorcluster)  [unwired: 1 out]
    n294 = call "AnemoASCIIConversion.vi"("Input string (from RS232)"=w707) -> ("Data out"=w706:T21)
    n295 = shared-variable ".\\SharedVars.lvlib\\AnemometerData"(w706) -> ()  [unwired: 1 in, 1 out]
    n296 = VISA Clear(VISA resource name=w710, error in (no error)=w709) -> (error out=w708:errorcluster)  [unwired: 1 out]
    n297 = shared-variable ".\\SharedVars.lvlib\\StopLabVIEW"() -> (w711:bool)  [unwired: 1 in, 1 out]
    n298 = node-c288() -> ()  [unwired: 1 in, 1 out]
  }
  n299 = timed-loop {
    timing: w91 -> [_]
    timing-out: [_] -> w90
    shift-right: [w722] -> _
    shift-left: T8 {"Elmo Operational"=FALSE, "Elmo Warning"=FALSE, "Elmo Fault"=FALSE, "Blade Homed"=FALSE, "Blade Homing"=FALSE, "HomePos (rad)"=0.0} ("Elmo State Cluster In") -> [w730]
    shift-right: [w721] -> _
    shift-left: T8 {"Elmo Operational"=FALSE, "Elmo Warning"=FALSE, "Elmo Fault"=FALSE, "Blade Homed"=FALSE, "Blade Homing"=FALSE, "HomePos (rad)"=0.0} ("Elmo State Cluster In") -> [w728]
    shift-right: [w720] -> _
    shift-left: T8 {"Elmo Operational"=FALSE, "Elmo Warning"=FALSE, "Elmo Fault"=FALSE, "Blade Homed"=FALSE, "Blade Homing"=FALSE, "HomePos (rad)"=0.0} ("Elmo State Cluster In") -> [w726]
    stop <- w747 stop-if-true
    # "TO DO:\nOnly allow home button when OP\nClear homing state when not in OP\nCheck if home pos (zero) remains consitent while drive is on/off and LabVIEW is on/off\nSet setpoint to zero when not homed"
    # "used in ctrl loop"
    # "used in ctrl loop"
    # "used in ctrl loop"
    # "Axis No. 3"
    # "Axis No. 2"
    # "Axis No. 1"
    # "State logic"
    n300 = node-c288() -> (→"State logic late?":bool)  [unwired: 1 in]
    n301 = shared-variable ".\\SharedVars.lvlib\\IOSignals"() -> (w719:T11)  [unwired: 1 in, 1 out]
    n302 = call "AccelnetInterface.vi"("Enable"="Enable Accelnet", "Clear Faults"="Clear Accelnet Faults", "IO Signals"=w719) -> ("Control word"=w742:u16, "Accelnet State"=w746:T22)  [unwired: 7 in]
    "Gen ctrl word" <- w742
    n303 = call "ElmoInterface.vi"("Elmo State Cluster In"=w730, "Axis No."=u32 1, "IO Signals"=w719, "Enable"="Enable Pitch Actuators (x3)", "Clear faults"="Clear Pitch Actuator Faults (x3)", "Home"="Home Blades (x3)") -> ("Elmo State Cluster Out"=w722:T8, "State String"=→"Pitch Axis 1 State":string, "Control word"=w739:u16)  [unwired: 7 in]
    "Pitch axis 1 ctrl word" <- w739
    n304 = call "ElmoInterface.vi"("Elmo State Cluster In"=w728, "Axis No."=u32 2, "IO Signals"=w719, "Enable"="Enable Pitch Actuators (x3)", "Clear faults"="Clear Pitch Actuator Faults (x3)", "Home"="Home Blades (x3)") -> ("Elmo State Cluster Out"=w721:T8, "State String"=→"Pitch Axis 2 State":string, "Control word"=w736:u16)  [unwired: 7 in]
    "Pitch axis 2 ctrl word" <- w736
    n305 = call "ElmoInterface.vi"("Elmo State Cluster In"=w726, "Axis No."=u32 3, "IO Signals"=w719, "Enable"="Enable Pitch Actuators (x3)", "Clear faults"="Clear Pitch Actuator Faults (x3)", "Home"="Home Blades (x3)") -> ("Elmo State Cluster Out"=w720:T8, "State String"=→"Pitch Axis 3 State":string, "Control word"=w735:u16)  [unwired: 7 in]
    "Pitch axis 3 ctrl word" <- w735
    n306 = Unbundle By Name(w746) -> ("State String"=→"Main generator state":string, "Accelnet Warning"=→"Generator Warning":bool, "Accelnet Fault"=→"Generator Fault":bool, "Accelnet Operational"=w737:bool)
    "Generator Operational" <- w737
    n307 = shared-variable "NI-cRIO-9036-01B82934\\EtherCAT Master\\MainGen\\Receive PDO 6 CSV-Control word"(w742) -> ()  [unwired: 1 in, 1 out]
    n308 = shared-variable ".\\SharedVars.lvlib\\PitchAxis2State"(w721) -> ()  [unwired: 1 in, 1 out]
    n309 = shared-variable "NI-cRIO-9036-01B82934\\EtherCAT Master\\PitchBlade2\\Outputs-Control word"(w736) -> ()  [unwired: 1 in, 1 out]
    n310 = shared-variable ".\\SharedVars.lvlib\\PitchAxis1State"(w722) -> ()  [unwired: 1 in, 1 out]
    n311 = shared-variable "NI-cRIO-9036-01B82934\\EtherCAT Master\\PitchBlade1\\Outputs-Control word"(w739) -> ()  [unwired: 1 in, 1 out]
    n312 = shared-variable ".\\SharedVars.lvlib\\PitchAxis3State"(w720) -> ()  [unwired: 1 in, 1 out]
    n313 = shared-variable "NI-cRIO-9036-01B82934\\EtherCAT Master\\PitchBlade3\\Outputs-Control word"(w735) -> ()  [unwired: 1 in, 1 out]
    n314 = shared-variable ".\\SharedVars.lvlib\\GeneratorOn"(w737) -> ()  [unwired: 1 in, 1 out]
    n315 = shared-variable ".\\SharedVars.lvlib\\StopLabVIEW"() -> (w747:bool)  [unwired: 1 in, 1 out]
    n316 = node-c288() -> ()  [unwired: 1 in, 1 out]
  }
  n317 = timed-loop {
    timing: w87 -> [_]
    timing-out: [_] -> w86
    tunnel: w84 -> [w798]
    i -> [w793]
    stop <- w799 stop-if-true
    # "Data recording to RT buffer"
    n318 = node-c288() -> (→"FIFO Loop Late?":bool)  [unwired: 1 in]
    n319 = shared-variable ".\\SharedVars.lvlib\\IOSignals"() -> (w796:T11)  [unwired: 1 in, 1 out]
    n320 = shared-variable ".\\SharedVars.lvlib\\GenCtrlMS"() -> (w773:T19)  [unwired: 1 in, 1 out]
    n321 = shared-variable ".\\SharedVars.lvlib\\PitchCtrlMS"() -> (w772:T20)  [unwired: 1 in, 1 out]
    n322 = shared-variable ".\\SharedVars.lvlib\\RoscoPairs"() -> (w777:T9)  [unwired: 1 in, 1 out]
    n323 = call "FileWriteTiming.vi"("Loop counter"=w793, "WriteData"="Start / Stop Run") -> ("Write counter"=w792:i32, "Time (s)"=w775:dbl)  [unwired: 8 in]
    n324 = shared-variable ".\\SharedVars.lvlib\\WriteData"("Start / Stop Run") -> ()  [unwired: 1 in, 1 out]
    n325 = shared-variable ".\\SharedVars.lvlib\\GenVelocitySetpoint_radps"() -> (w763:dbl)  [unwired: 1 in, 1 out]
    n326 = Unbundle By Name(w777) -> ("TorqueSetpoint_Nm.Value"=w767:dbl, "BladePitchSetpoint_rad.Value"=w766:dbl)  [unwired: 3 out]
    n327 = Unbundle By Name(w772) -> ("Blade pitch operating mode"=w768:T4)
    n328 = Unbundle By Name(w773) -> ("Generator operating mode"=w771:T2)
    n329 = shared-variable ".\\SharedVars.lvlib\\GenTorqueSetpoint_Nm"() -> (w765:dbl)  [unwired: 1 in, 1 out]
    n330 = Unbundle By Name(w796) -> ("anemoRefU_m_s"=w752:dbl, "torqueSensor (Nm)"=w753:dbl, "towerTopFx (N)"=w761:dbl, "towerTopFy (N)"=w760:dbl, "towerBotMy (Nm)"=w759:dbl, "nacelleAccX (m/s2)"=w758:dbl, "nacelleAccY (m/s2)"=w757:dbl, "nacelleAccZ (m/s2)"=w756:dbl, "mainGenVelocity (rad/s)"=w795:dbl, "motorCurrentTorq (Nm)"=w794:dbl, "mainGenStatus"=w790:u16, "pitch1Position (rad)"=w789:dbl, "pitch1Velocity (rad/s)"=w788:dbl, "pitch1Status"=w786:u16, "pitch2Position (rad)"=w785:dbl, "pitch2Velocity (rad/s)"=w784:dbl, "pitch2Status"=w783:u16, "pitch3Position (rad)"=w781:dbl, "pitch3Velocity (rad/s)"=w780:dbl, "pitch3Status"=w779:u16)
    n331 = shared-variable ".\\SharedVars.lvlib\\PitchSetpoint_rad"() -> (w764:dbl)  [unwired: 1 in, 1 out]
    n332 = shared-variable ".\\SharedVars.lvlib\\FanSetpoint_unit"() -> (w755:dbl[])  [unwired: 1 in, 1 out]
    n333 = To Double Precision Float(number=w792) -> (double precision float=w797:dbl)
    n334 = Index Array(array=w755, index=0) -> (element=w751:dbl)
    n335 = To Double Precision Float(number=w786) -> (double precision float=w787:dbl)
    n336 = To Double Precision Float(number=w783) -> (double precision float=w782:dbl)
    n337 = To Double Precision Float(number=w779) -> (double precision float=w778:dbl)
    n338 = To Double Precision Float(number=w771) -> (double precision float=w770:dbl)
    n339 = To Double Precision Float(number=w768) -> (double precision float=w769:dbl)
    n340 = To Double Precision Float(number=w790) -> (double precision float=w791:dbl)
    n341 = Bundle By Name(cluster=T6 {"dataTime_s"=0.0, "dataLoopCounter"=0.0, "anemoRefU_m_s"=0.0, "anemoRefV_m_s"=0.0, "anemoRefW_m_s"=0.0, "rotorTorque_Nm"=0.0, "towerTopFx_N"=0.0, "towerTopFy_N"=0.0, "towerBotMy_Nm"=0.0, "accelNacelleAx_m_s2"=0.0, "accelNacelleAy_m_s2"=0.0, "accelNacelleAz_m_s2"=0.0, "genSpeed_rad_s"=0.0, "genTorque_Nm"=0.0, "genStatus"=0.0, "pitch1Position_rad"=0.0, "pitch1Velocity_rad_s"=0.0, "pitch1Status"=0.0, "pitch2Position_rad"=0.0, "pitch2Velocity_rad_s"=0.0, "pitch2Status"=0.0, "pitch3Position_rad"=0.0, "pitch3Velocity_rad_s"=0.0, "pitch3Status"=0.0, "genUserOpMode"=0.0, "pitchUserOpMode"=0.0, "torqueSetpointRosco_Nm"=0.0, "pitchSetpointRosco_rad"=0.0, "fan1Setpt_%"=0.0, "genTorqueSetpointActual_Nm"=0.0, "pitchSetpointActual_rad"=0.0, "genVelSetpoint_radps"=0.0, "genPosition_rad"=0.0, "towerTopFz_N"=0.0, "towerTopMx_Nm"=0.0, "towerTopMy_Nm"=0.0, "towerTopMz_Nm"=0.0} ("SwapIn"), "dataTime_s"=w775, "dataLoopCounter"=w797, "anemoRefU_m_s"=w752, "rotorTorque_Nm"=w753, "towerTopFx_N"=w761, "towerTopFy_N"=w760, "towerBotMy_Nm"=w759, "accelNacelleAx_m_s2"=w758, "accelNacelleAy_m_s2"=w757, "accelNacelleAz_m_s2"=w756, "genSpeed_rad_s"=w795, "genTorque_Nm"=w794, "genStatus"=w791, "pitch1Position_rad"=w789, "pitch1Velocity_rad_s"=w788, "pitch1Status"=w787, "pitch2Position_rad"=w785, "pitch2Velocity_rad_s"=w784, "pitch2Status"=w782, "pitch3Position_rad"=w781, "pitch3Velocity_rad_s"=w780, "pitch3Status"=w778, "genUserOpMode"=w770, "pitchUserOpMode"=w769, "torqueSetpointRosco_Nm"=w767, "pitchSetpointRosco_rad"=w766, "fan1Setpt_%"=w751, "genTorqueSetpointActual_Nm"=w765, "pitchSetpointActual_rad"=w764, "genVelSetpoint_radps"=w763) -> (w762:T6)
    n342 = call "FileBuffer.vi"("Write Data"="Start / Stop Run", "FileDataChannel"=w762, "Refnum in"=w798) -> ("dataTime_s"=w774:dbl, "# elements"=→"#RT FIFO":u32)  [unwired: 7 in]
    "Exp. Time MS (s)" <- w774
    n343 = shared-variable ".\\SharedVars.lvlib\\ExpTime_s"(w774) -> ()  [unwired: 1 in, 1 out]
    n344 = shared-variable ".\\SharedVars.lvlib\\StopLabVIEW"() -> (w799:bool)  [unwired: 1 in, 1 out]
    n345 = node-c288() -> ()  [unwired: 1 in, 1 out]
  }
  n346 = while {
    shift-right: [w812] -> _
    shift-left: _ -> [w813]
    shift-right: [w818] -> _
    shift-left: FALSE -> [w819]
    shift-right: [w821] -> w93
    shift-left: errorcluster {"status"=FALSE, "code"=0, "source"=""} ("error out") -> [w820]
    tunnel: "focalC1" -> [w815]
    tunnel: w97 -> [w808]
    tunnel: w84 -> [w816]
    tunnel: w50 -> [w807]
    tunnel: w49 -> [w806]
    stop <- w823 stop-if-true
    # "Access the file system every 200ms, writing buffered data. This ensures that the \"slow\" file system is not accessed too often."
    # "Create directory if doesnt exist"
    # "File access loop (non RT loop, read from RT buffer)"
    n347 = Wait (ms)(milliseconds to wait=u32 200) -> ()  [unwired: 1 out]
    n348 = shared-variable ".\\SharedVars.lvlib\\WriteData"() -> (w809:bool)  [unwired: 1 in, 1 out]
    n349 = call "CheckFIleWriteStatus.vi"("WriteDataButtonVal"=w809, "WritePrevVal"=w819, "Refnum in"=w813, "Base filename"="Base filename", "File path"=path "C:/focal-data") -> ("File Name"=→"Output file Name":string, "Refnum out"=w812:refnum<k34>, "WriteCurrentVal"=w818:bool)  [unwired: 4 in]
    n350 = call "WriteToFile-v3.vi"("Refnum in"=w812, "Group Name"=w815, "IO Names"=w808, "rt fifo"=w816, "Write?"=w809, "error in (no error)"=w820, "ConstNames"=w807, "ConstValues"=w806) -> ("Writing to file"=→"Writing":bool, "error out"=w821:errorcluster)  [unwired: 5 in, 1 out]
    n351 = shared-variable ".\\SharedVars.lvlib\\StopLabVIEW"() -> (w824:bool)  [unwired: 1 in, 1 out]
    n352 = Or(x=w821, y=w824) -> (x .or. y?=w823:bool)
  }
  n353 = node-c288(w86) -> ()  [unwired: 1 out]
  n354 = node-c288(w11) -> ()  [unwired: 1 out]
  n355 = node-c288(w90) -> ()  [unwired: 1 out]
  n356 = node-c288(w25) -> ()  [unwired: 1 out]
  n357 = node-c288(w70) -> ()  [unwired: 1 out]
  n358 = node-c288(w79) -> ()  [unwired: 1 out]
  n359 = call <vilib>:"Simple Error Handler.vi"("error in (no error)"=w77) -> ()  [unwired: 4 in, 5 out]
  n360 = call <vilib>:"Simple Error Handler.vi"("error in (no error)"=w93) -> ()  [unwired: 4 in, 5 out]
